vi "WSVCAP SHL FPGA TL Top Level.vi"() -> ()   [LabVIEW 2017]
uses:
  Type Defs/WSVCAP SHL State.ctl
  Type Defs/WSVCAP SHL Transaction Enum.ctl
  Type Defs/WSVCAP SHL Communication Loop State.ctl
  Type Defs/WSVCAP SHL FIFO Operation Enum.ctl
  Type Defs/WSVCAP SHL Operation Step Enum.ctl
  Type Defs/WSVCAP SHL Procedure Step Enum.ctl
  Type Defs/WSVCAP SHL Transaction Step Enum.ctl
  <vilib>/Platform/TimedLoop/XDataNode/timing_clust.ctl
  <vilib>/Platform/TimedLoop/XDataNode/nitl_modes.ctl
  <vilib>/Platform/TimedLoop/XDataNode/wakeup.ctl
  WSVCAP Shell FPGA Low Level/WSVCAP SHL FPGA LL RFFE Debug Global.vi
  WSVCAP Shell FPGA Low Level/WSVCAP SHL FPGA LL I2C Debug Global.vi
  <vilib>/Platform/TimedLoop/XDataNode/XDataNode.xnode
  <vilib>/Platform/TimedLoop/XDataNode/XDNodeRunTimeDep.lvlib
panel:
  in  "UUT Set":u8=8
  in  "Stop Cycle":bool
  out "Cycle Count":u64
  in  "Socket Mask":u64=1 format="%012x"
  in  "Display CH (1-48)":i32=1 min=1 max=48 step=1
  out "Status":i32
  out "Read Data":u64
  in  "Transaction":T1
  in  "Bytes to Write":u8=8
  in  "Sub Address":u8=1 format="%02x"
  in  "Ack Read Status":bool
  out "Read Status Flag":bool
  in  "Exit":bool
  out "Waveform Chart":cluster{i16, i16, i16, i16}(graph)
  in  "Wait Ticks":u32=20
  in  "Slave Address":u8=1 format="%02x"
  in  "Bytes to Read":u8=8
  in  "Start":bool
  in  "Cmd":T2
  in  "Ack Read":bool
  out "Read Flag":bool
  in  "Write Flag":bool
  in  "Write Data":u64
  # "Control"
  # "Configuration Parameters"
  # "Host Data Transfer"
  # "Command Type"
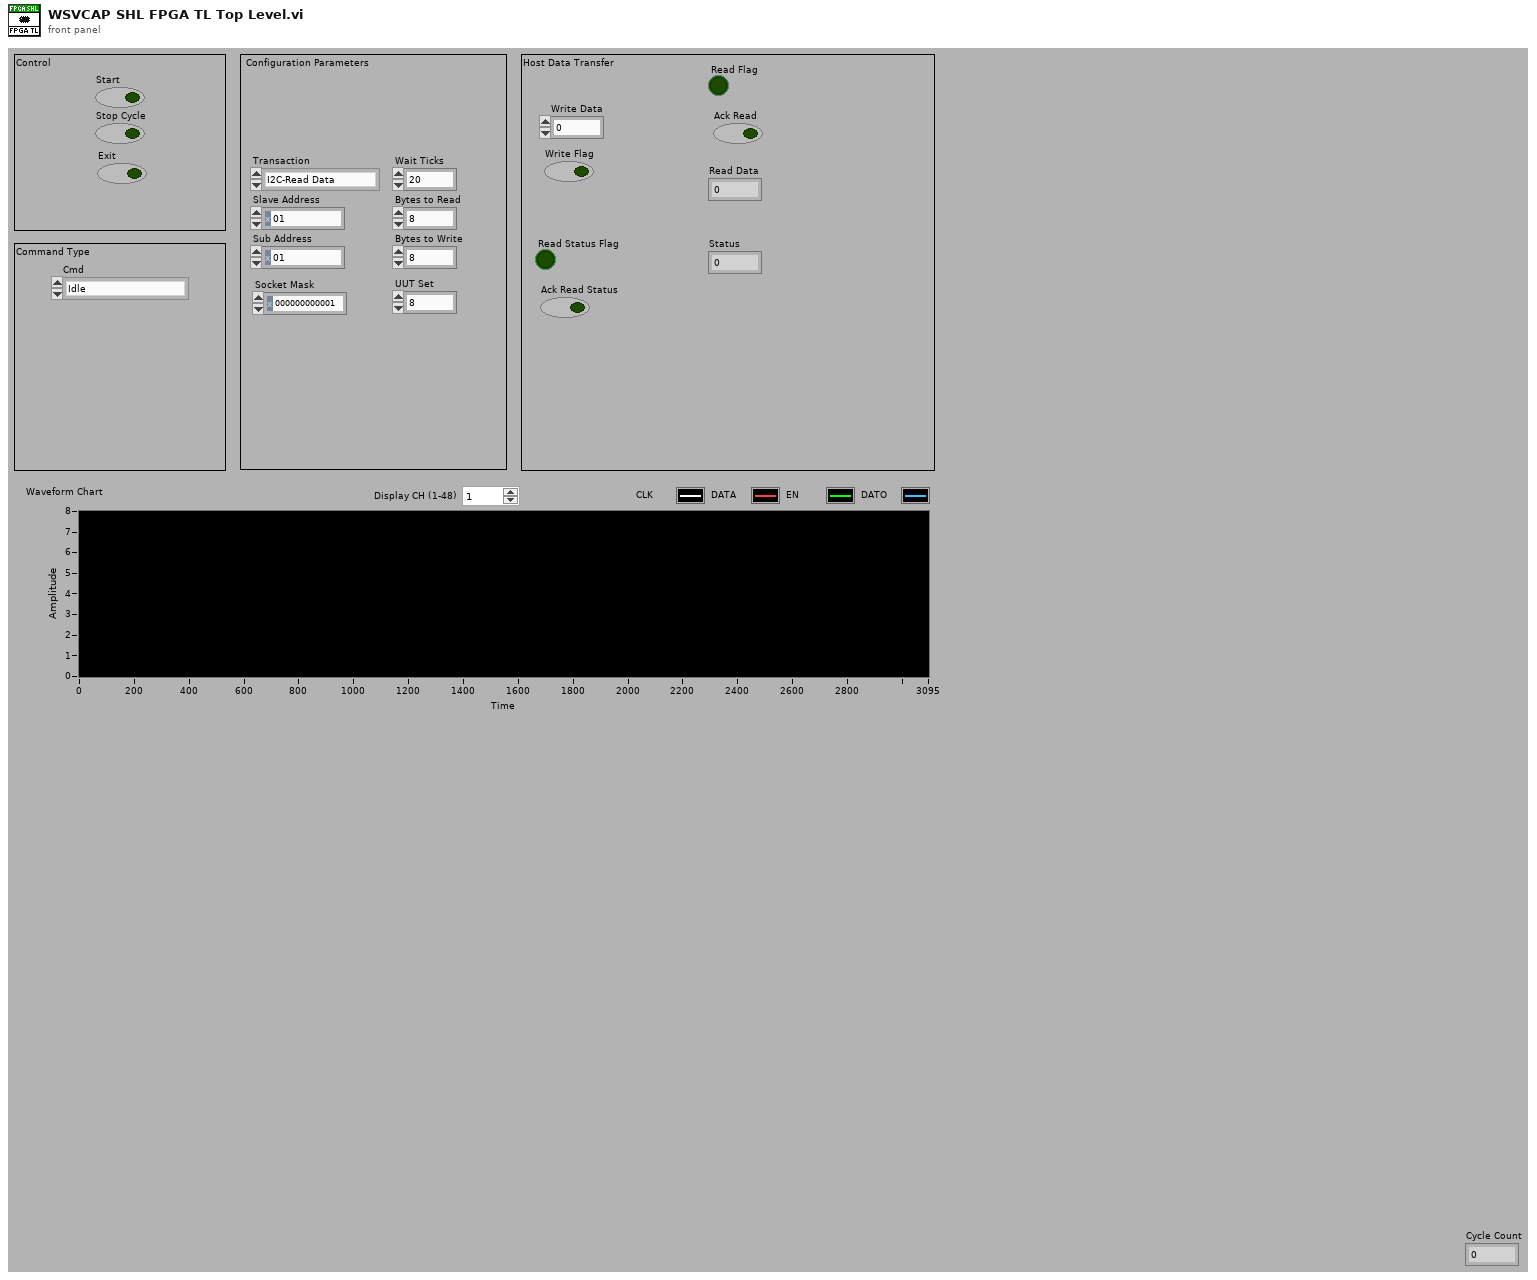
[diagram p1: front panel]
types:
  T1 = typedef "WSVCAP SHL Transaction Enum.ctl" = enum16{"I2C-Read Data", "I2C-Write Data", "RFFE-Ext Write", "RFFE-Ext Read"}
  T2 = typedef "WSVCAP SHL State.ctl" = enum8{"Idle", "Transfer Data"}
  T3 = typedef "WSVCAP SHL Communication Loop State.ctl" = enum8{"Idle", "Initialize", "Pre-Transmission", "Transmit Data", "Post Transmition", "Operation Complete"}
  T4 = typedef "WSVCAP SHL FIFO Operation Enum.ctl" = enum16{"Create FIFO/Memory", "Get Write FIFO Status", "Get Read FIFO Status", "Put Element in Write", "Put Element in Read", "Get Element from Write", "Get Element from Read"}
  T5 = typedef "WSVCAP SHL Procedure Step Enum.ctl" = enum16{"I2C Start/Stop - 1: Set Clock Low", "I2C Start/Stop - 2: Wait", "I2C Start/Stop - 3: Set Data I", "I2C Start/Stop - 4: Wait", "I2C Start/Stop - 5: Set Clock High", "I2C Start/Stop - 6: Wait", "I2C Start/Stop - 7: Set Data II", "I2C Start/Stop - 8: Wait", "I2C Start/Stop - 9: Set Clock Low", "I2C Start/Stop - 10: Wait", "I2C Read ACK - 1: Set Clock High", "I2C Read ACK - 2: Wait", "I2C Read ACK - 3: Read ACK Bit", "I2C Read ACK - 4: Wait", "I2C Read ACK - 5: Set Clock Low", "I2C Read ACK - 6: Wait", "I2C Write ACK - 1: Write ACK Bit", "I2C Write ACK - 2: Wait", "I2C Write ACK - 3: Set Clock High", "I2C Write ACK - 4: Wait", "I2C Write ACK - 5: Set Clock Low", "I2C Write ACK - 6: Wait", "I2C Write ACK - 7: Set Data Low", "I2C Send Add - 1: Reset Bits Remaining", "I2C Send Add - 2: Set Data Bit", "I2C Send Add - 3: Wait", "I2C Send Add - 4: Set Clock High", "I2C Send Add - 5: Wait", "I2C Send Add - 6: Set Clock Low", "I2C Send Add - 7: Wait", "I2C Send Add - 8: Check Bits Remaining", "I2C Send Data - 1: Reset Bits Remaining", "I2C Send Data - 2: Load Write Bit from FIFO", "I2C Send Data - 3: Set Data Bit", "I2C Send Data - 4: Wait", "I2C Send Data - 5: Set Clock High", "I2C Send Data - 6: Wait", "I2C Send Data - 7: Set Clock Low", "I2C Send Data - 8: Wait", "I2C Send Data - 9: Check Bits Remaining", "I2C Receive Data - 1: Reset Bits Remaining", "I2C Receive Data - 2: Wait", "I2C Receive Data - 3: Set Clock High", "I2C Receive Data - 4: Wait", "I2C Receive Data - 5: Read Data Bit", "I2C Receive Data - 6: Wait", "I2C Receive Data - 7: Set Clock Low", "I2C Receive Data - 8: Wait", "I2C Receive Data - 9: Check Bits Remaining", "RFFE Send SSC - 1:Set Low", "RFFE Send SSC - 2:Wait", "RFFE Send SSC - 3:Set SDA High", "RFFE Send SSC - 4:Wait", "RFFE Send SSC - 5:Set SDA Low", "RFFE Send SSC - 6:Wait", "RFFE Send Data - 1:Set SCL High", "RFFE Send Data - 2:Wait", "RFFE Send Data - 3:Set SCL Low", "RFFE Send Data - 4:Wait", "RFFE Send Data - 5:Set SCL High (P)", "RFFE Send Data - 6:Wait", "RFFE Send Data - 7:Set SCL Low (P)", "RFFE Send Data - 8:Wait", "RFFE Send Data - 9:Set SCL High (BP)", "RFFE Send Data - 10:Wait", "RFFE Send Data - 11:Set SCL Low (BP)", "RFFE Send Data - 12:Wait", "RFFE Receive Data - 1:Set SCL High", "RFFE Receive Data - 2:Wait", "RFFE Receive Data - 3:Set SCL Low", "RFFE Receive Data - 4:Wait", "RFFE Receive Data - 5:Set SCL High (BP)", "RFFE Receive Data - 6:Wait", "RFFE Receive Data - 7:Set SCL Low (BP)", "RFFE Receive Data - 8:Wait", "RFFE Wait CMD Delay - 1:Wait", "RFFE Clear Lines - 1:Clear"}
  T6 = typedef "WSVCAP SHL Operation Step Enum.ctl" = enum16{"I2C Send Slave Add - A: Send Start Sequence", "I2C Send Slave Add - B: Load Address Byte", "I2C Send Slave Add - C: Send Address Byte", "I2C Send Slave Add - D: Read Slave ACK", "I2C Send Sub Add - A: Load Sub Address", "I2C Send Sub Add - B: Send Address Byte", "I2C Send Sub Add - C: Read Slave ACK", "I2C Send Data - A: Get Byte from FIFO", "I2C Send Data - B: Send Data Byte", "I2C Send Data - C: Read Slave ACK", "I2C Send Data - D: Send Stop Sequence", "I2C Read Data - A: Load Bytes to Read", "I2C Read Data - B: Receive Byte", "I2C Read Data - C: Write Master ACK", "I2C Read Data - D: Send Stop Sequence", "RFFE Read Data - A: Send SSC", "RFFE Read Data - B: Send CMD Frame", "RFFE Read Data - C: Receive Byte", "RFFE Write Data - A: Send SSC", "RFFE Write Data - B: Send Data", "RFFE Write Data - C: Wait CMD Delay", "RFFE Write Data - D: Clear Lines"}
  T7 = typedef "WSVCAP SHL Transaction Step Enum.ctl" = enum16{"I2C Write - I:Send Slave Address", "I2C Write - II:Send Sub Address", "I2C Write - III:Send Data Bytes", "I2C Read - I:Send Slave Address (W)", "I2C Read - II:Send Sub Address", "I2C Read - III:Send Slave Address (R)", "I2C Read - IV:Read Data Bytes", "RFFE Ext Write - I.Write Data", "RFFE Ext Read - I:Read Data"}
  T8 = typedef "XDNodeRunTimeDep.lvlib/timing_clust.ctl" = cluster{"Expected End [f-1]":u64, "Actual End [f-1]":u64, "Finished Late? [f-1]":bool, "Expected End [i-1]":u64, "Actual End [i-1]":u64, "Finished Late? [i-1]":bool, "Expected Start [i]":u64, "Actual Start [i]":u64, "Expected Start [f]":u64, "Actual Start [f]":u64, "Source Name":string, "Structure Name":string, "Period":i64, "Deadline":i64, "Offset":i64, "Start":i64, "Priority":i32, "Timeout":i32, "Mode":T9, "Wakeup Reason":T10, "Error":errorcluster, "Source Type":string, "Secondary Source Type":string, "Global End Time":u64, "Global Start Time":u64, "Frame Duration":u64, "Iteration Duration":u64, "Assigned CPU":i32, "I/O Scan Engine Mode":u32}
  T9 = typedef "XDNodeRunTimeDep.lvlib/nitl_modes.ctl" = enum32{"No Change", "Process missed periods, maintain original phase", "Discard missed periods, maintain original phase", "Process missed periods, ignore original phase", "Discard missed periods, ignore original phase"}
  T10 = typedef "XDNodeRunTimeDep.lvlib/wakeup.ctl" = enum32{"Normal", "Aborted", "Asynchronous wakeup", "Timing source error", "Timed loop error", "Timeout"}
  T11 = typedef "WSVCAP SHL Transaction Cluster.ctl" = cluster{"Transaction":T1, "Write Byte":u8, "Write Bits Remaining":u8, "Read Bits Remaining":u8, "Read Bytes Remaining":u8, "Wait Ticks Remaining":u32, "Slave Address":u8, "Bytes to Read":u8, "Bytes to Write":u8, "Sub Address":u8, "Socket Mask":u64, "Write CMD [1-4]":u8, "Write Bit Index [0-39]":u8, "CMD Delay (Ticks)":u32, "Commands per Cycle [1-4]":u8, "CMD Length [1-48]":u8, "Cycle Count":u64, "Cycle Mode":bool, "CMD 1 Length (Bits)":u8, "CMD 2 Length (Bits)":u8, "CMD 3 Length (Bits)":u8, "CMD 4 Length (Bits)":u8, "CMD 1 Delay (Ticks)":u32, "CMD 2 Delay (Ticks)":u32, "CMD 3 Delay (Ticks)":u32, "CMD 4 Delay (Ticks)":u32, "CMD 1":u64, "CMD 2":u64, "CMD 3":u64, "CMD 4":u64, "Cycle CMD":u64, "Transaction Step":T7, "Operation Step":T6, "Procedure Step":T5, "Start Operation":bool, "Start Procedure":bool, "Procedure":T12, "Wait Ticks":u32, "UUT Set (0/1)":u8}
  T12 = typedef "WSVCAP SHL Procedure Enum.ctl" = enum16{"None", "I2C-Send Start/Stop Sequence", "I2C-Send Address Byte", "I2C-Send Data Byte", "I2C-Read ACK", "I2C-Receive Byte", "I2C-Write ACK", "RFFE-Clear Lines", "RFFE-Send SSC", "RFFE-Send Data", "RFFE-Receive Data", "RFFE-Wait CMD Delay"}
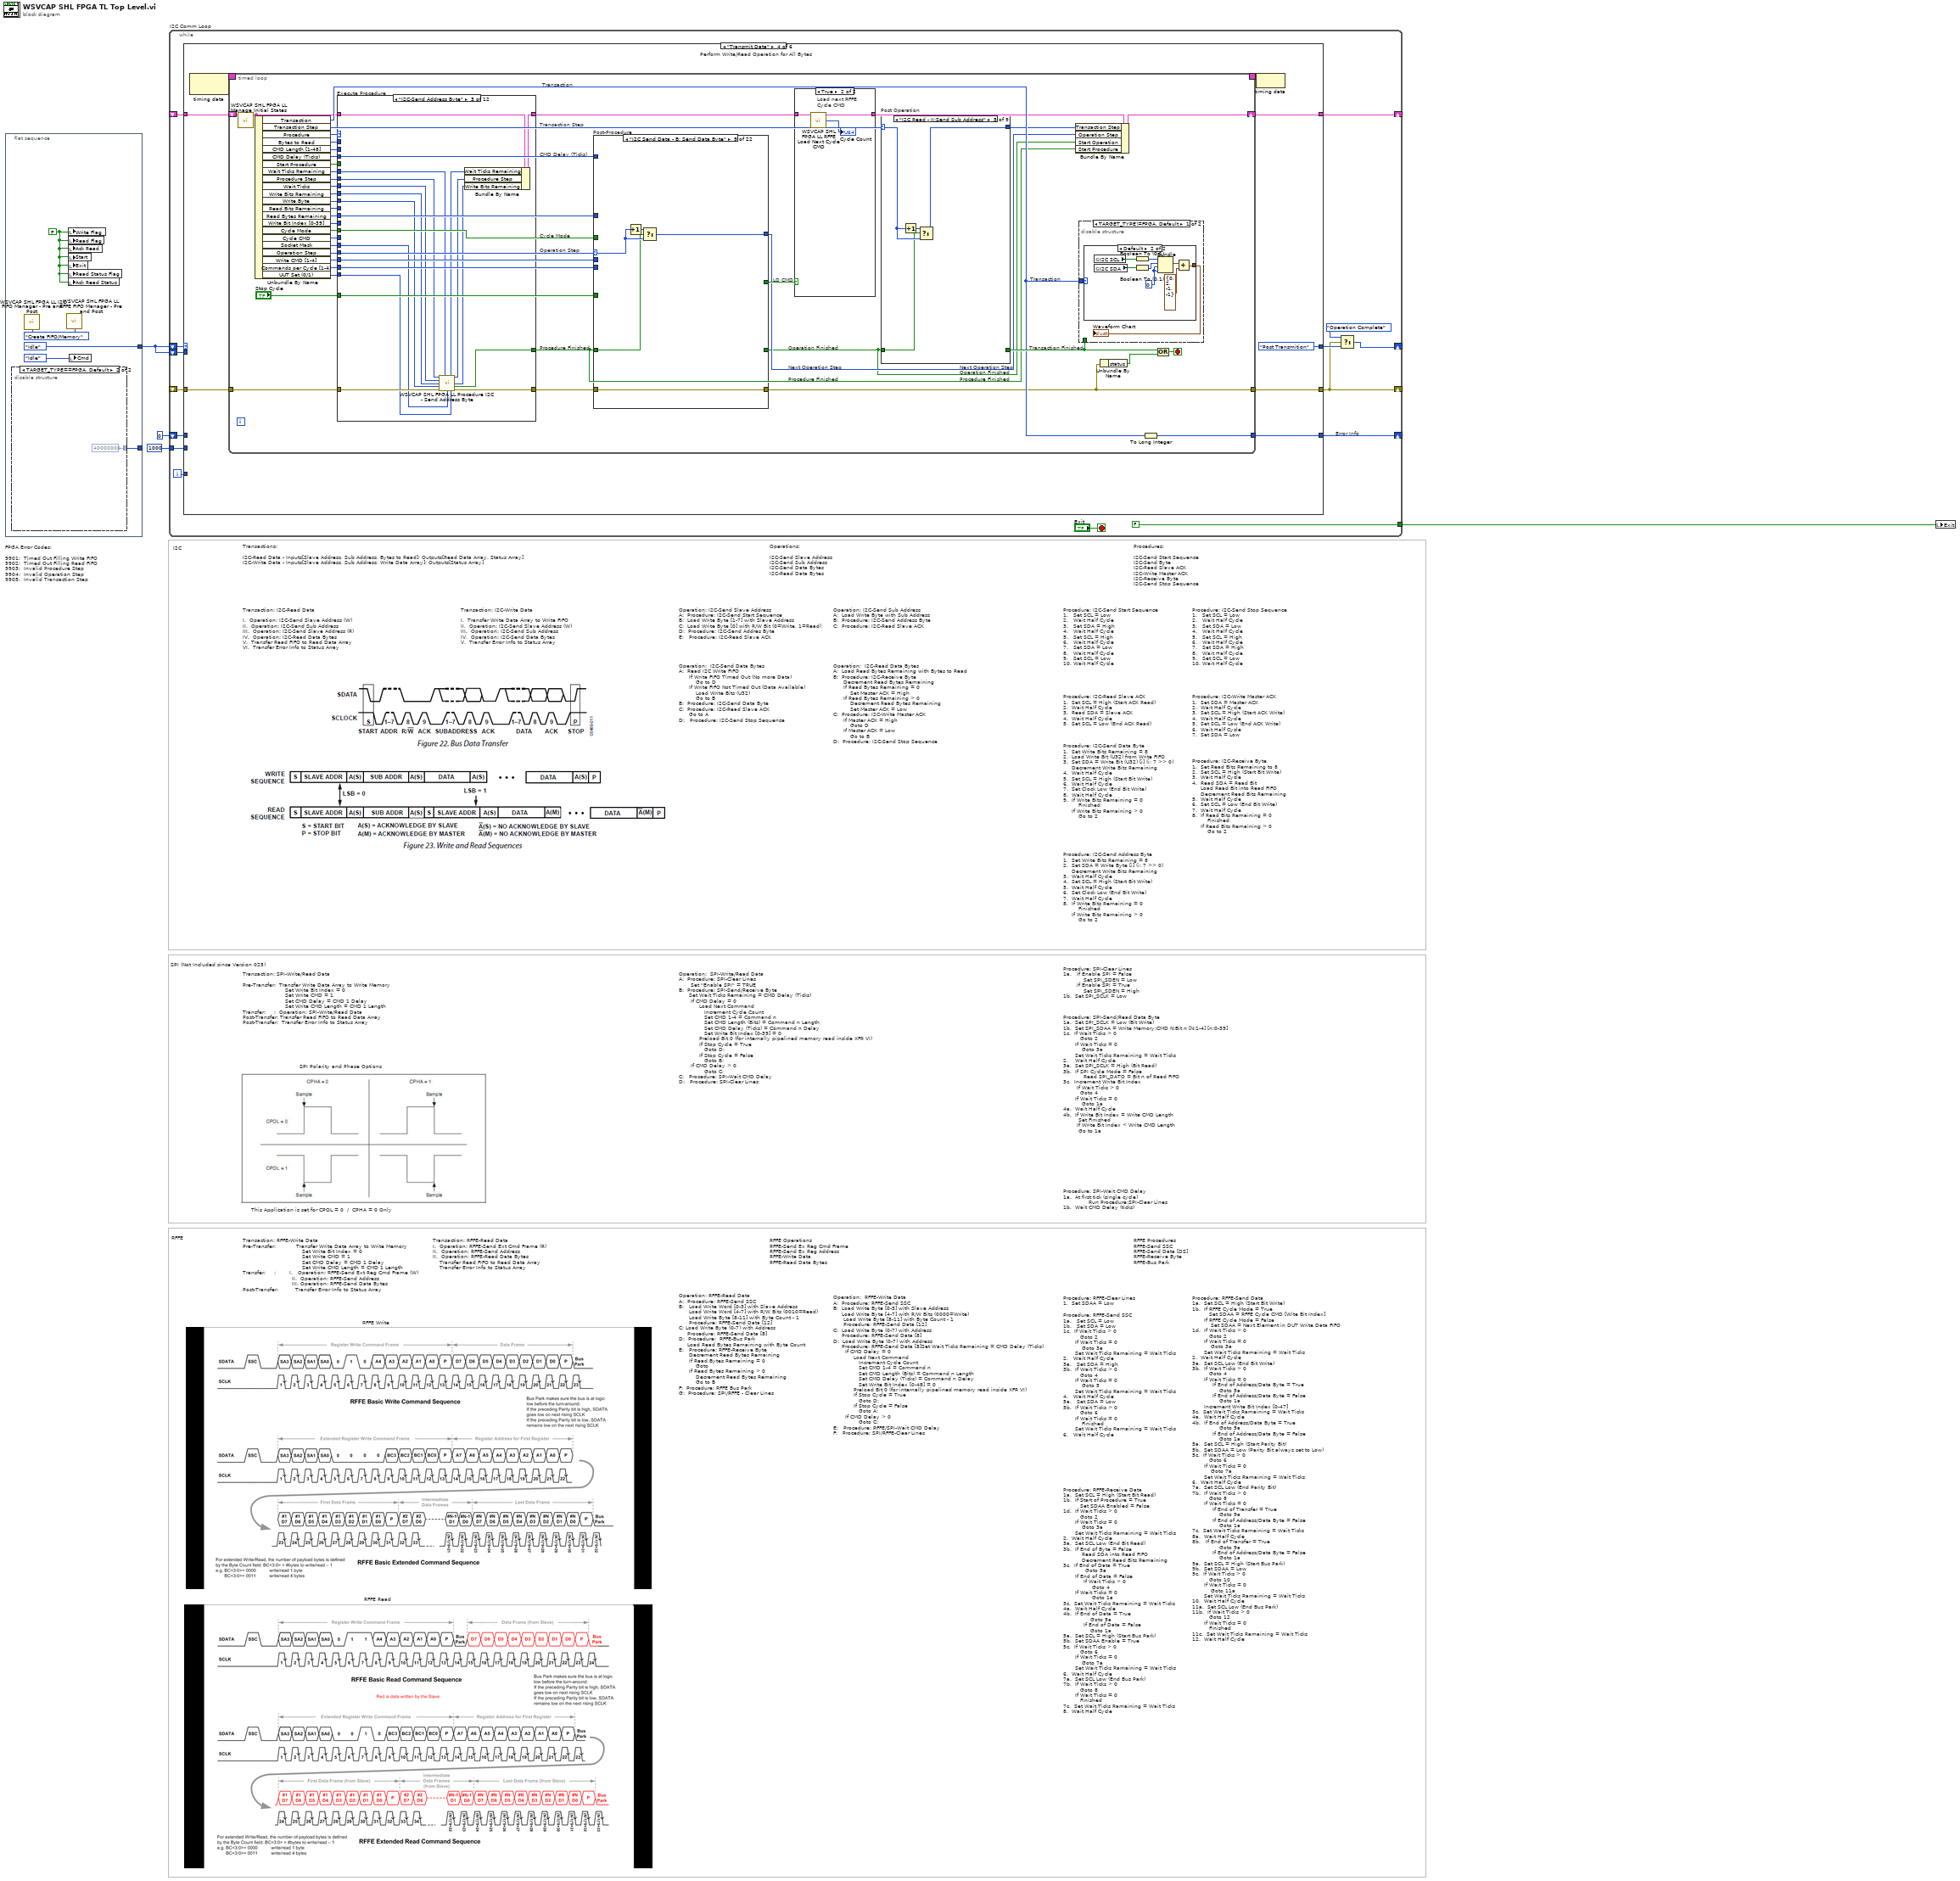
[diagram p0: block diagram]
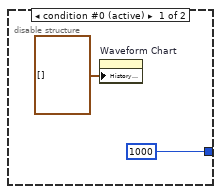
[diagram p2: hidden frame]
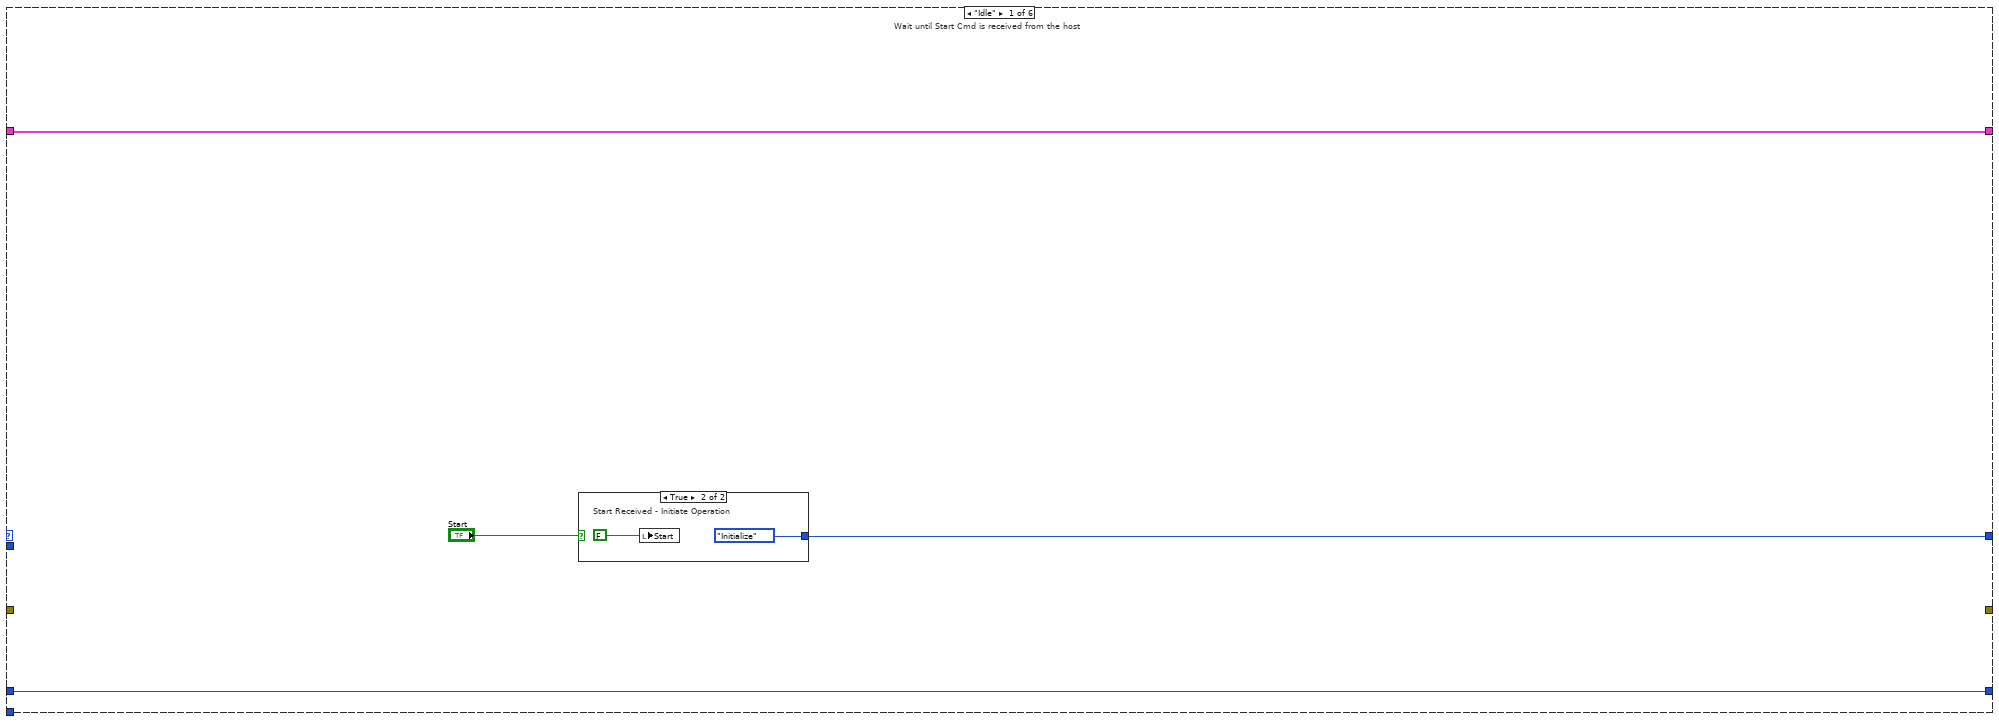
[diagram p3: hidden frame]
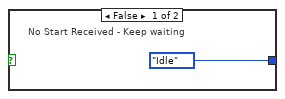
[diagram p4: hidden frame]
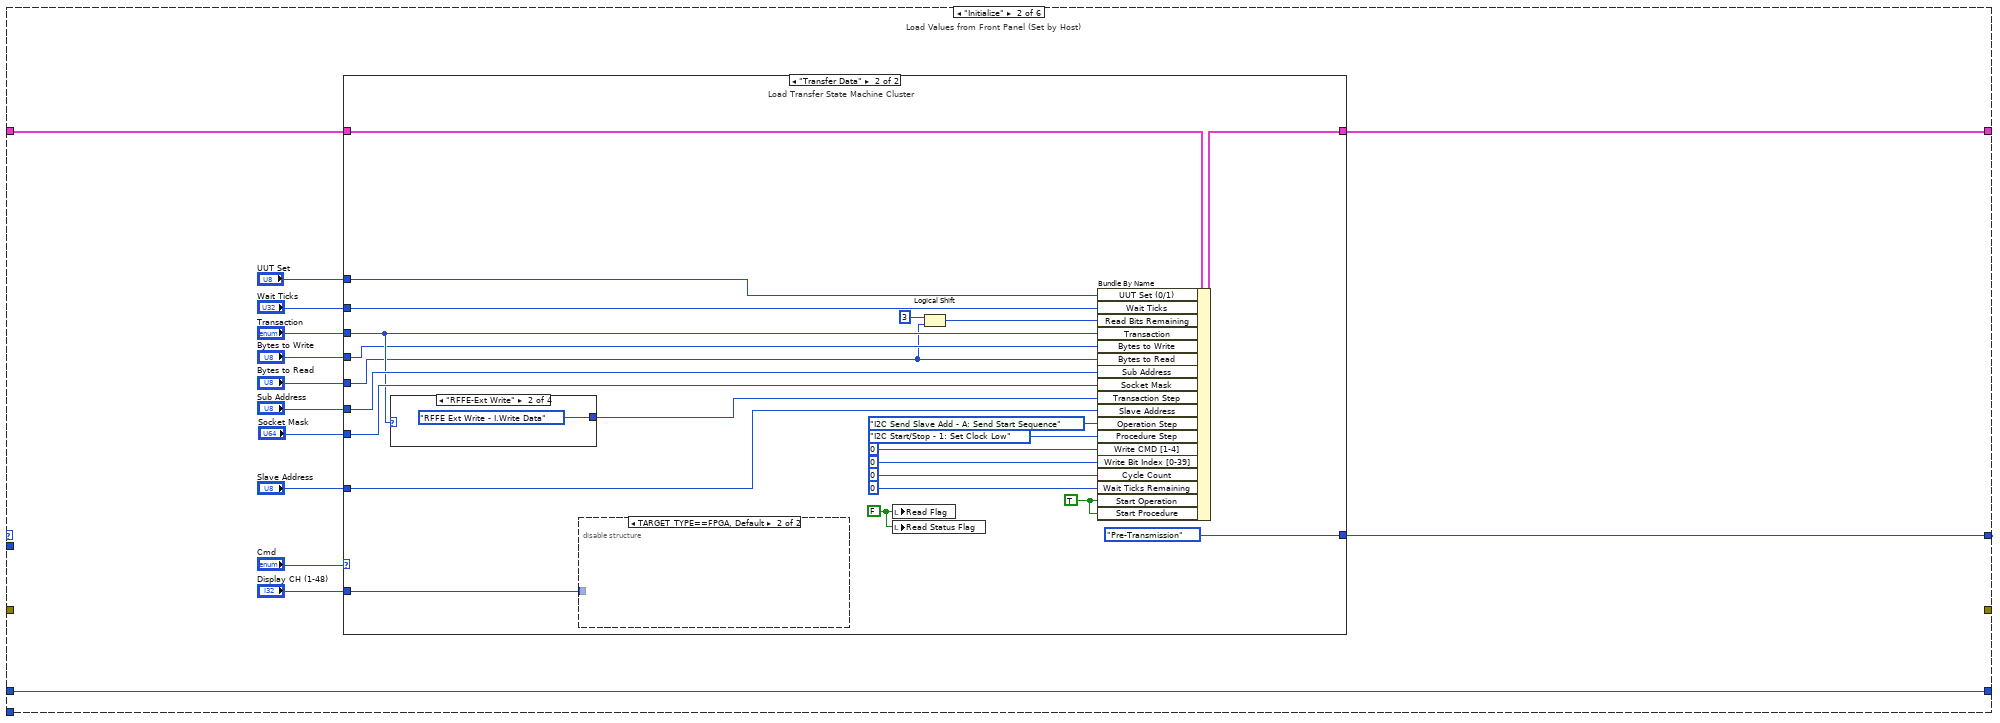
[diagram p5: hidden frame]
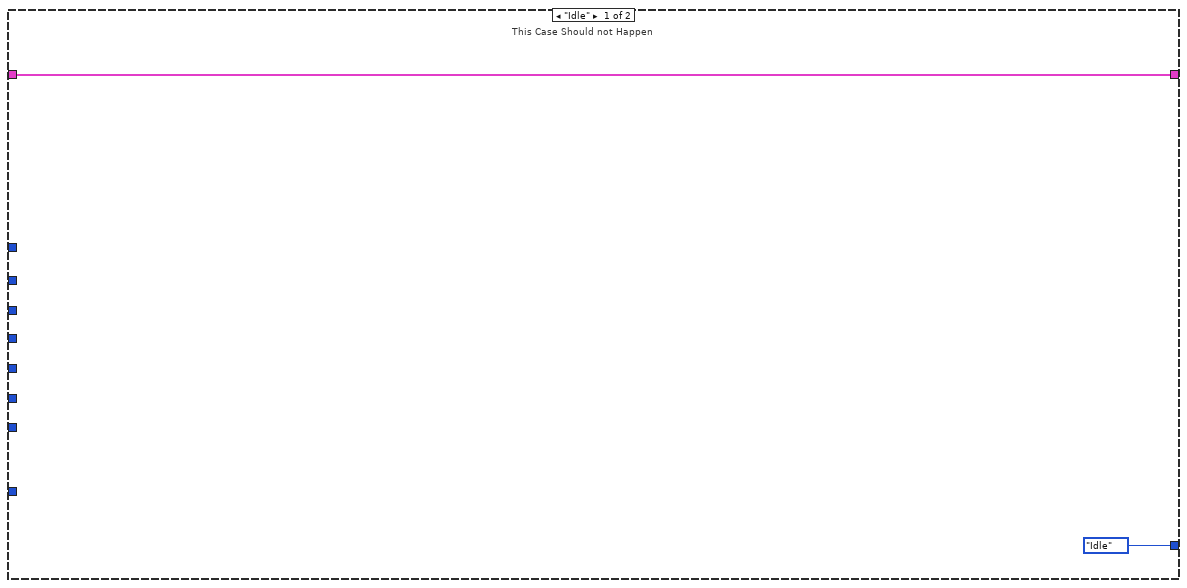
[diagram p6: hidden frame]
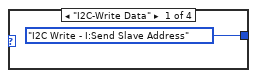
[diagram p7: hidden frame]
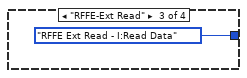
[diagram p8: hidden frame]
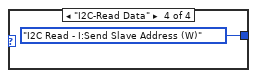
[diagram p9: hidden frame]
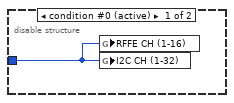
[diagram p10: hidden frame]
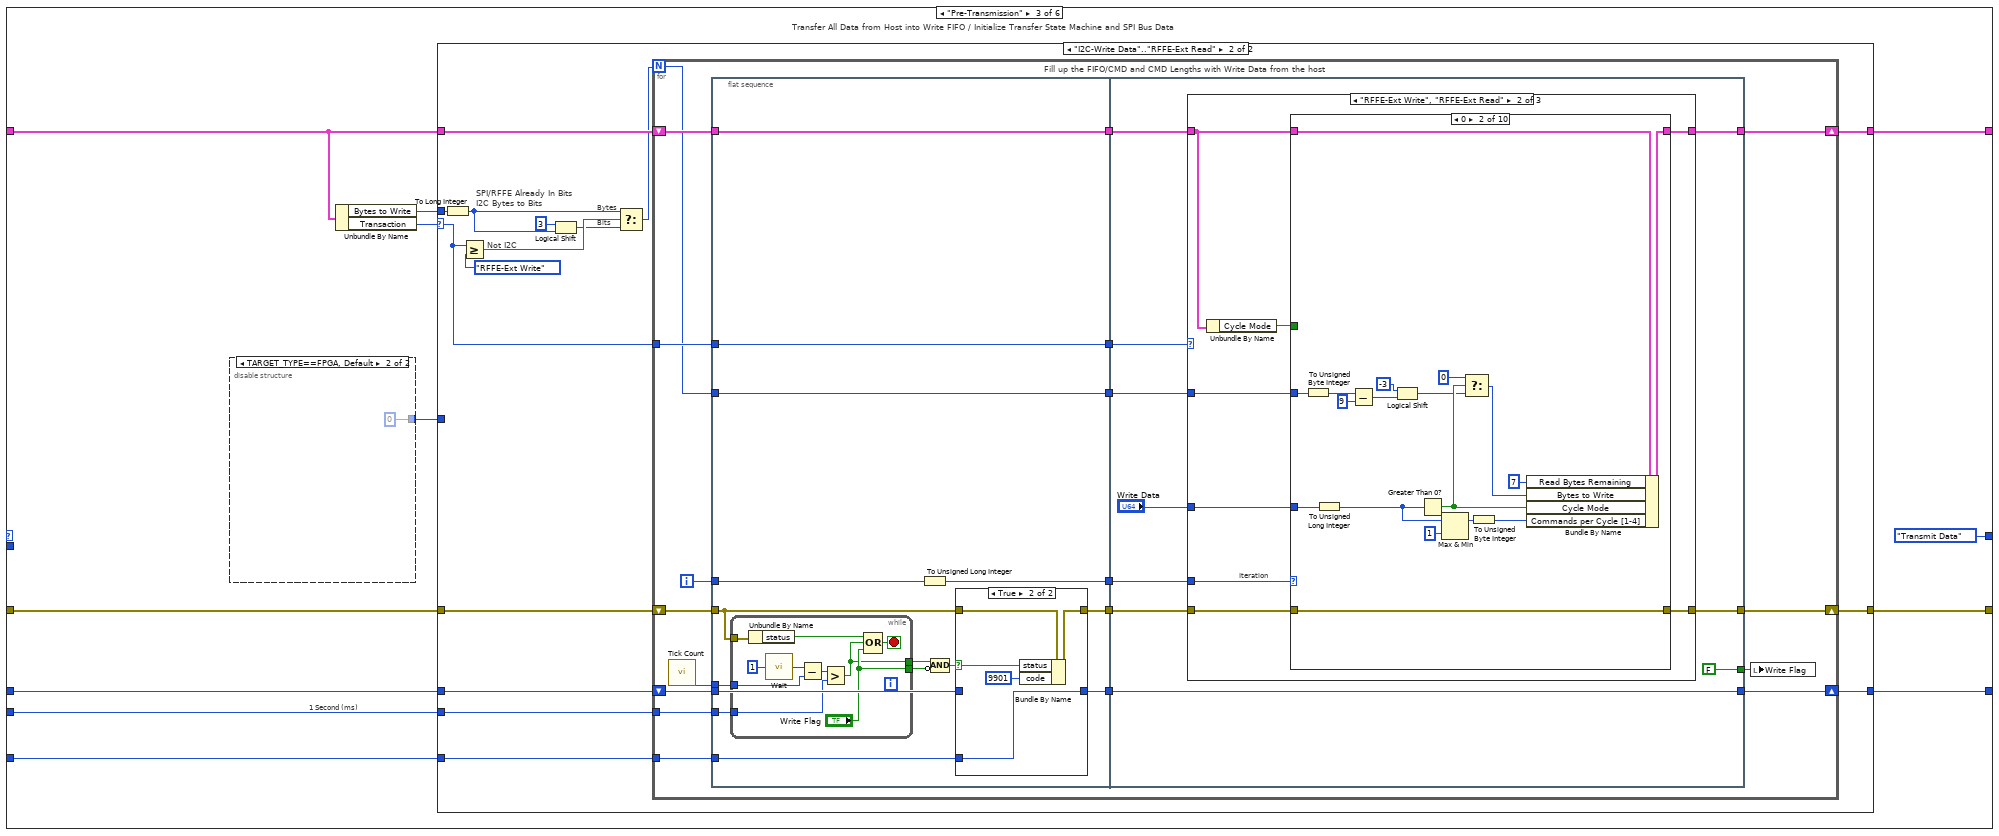
[diagram p11: hidden frame]
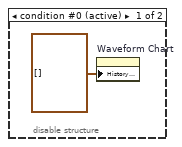
[diagram p12: hidden frame]
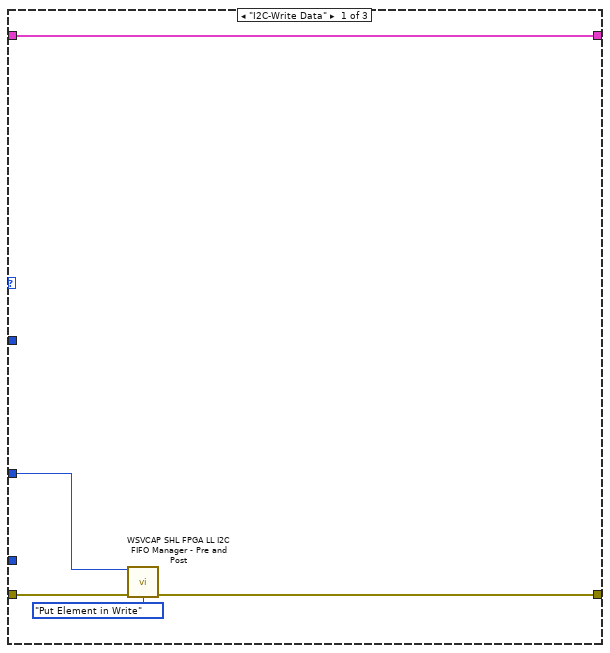
[diagram p15: hidden frame]
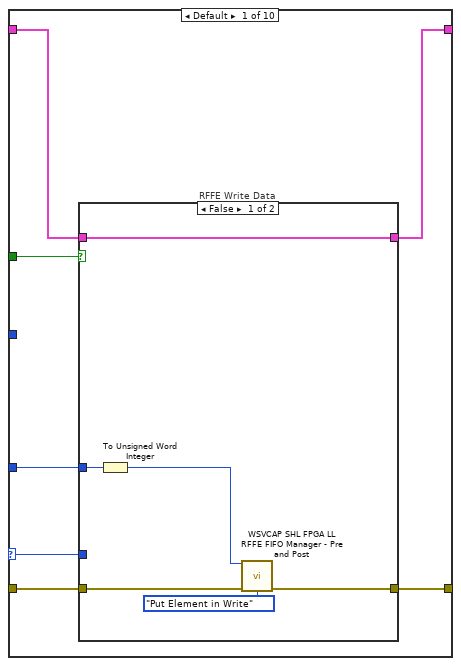
[diagram p16: hidden frame]
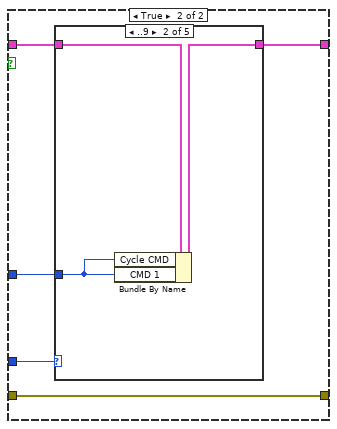
[diagram p17: hidden frame]
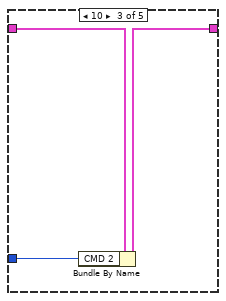
[diagram p19: hidden frame]
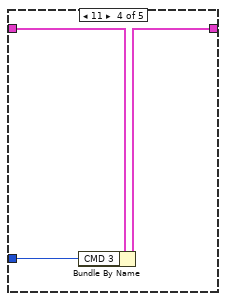
[diagram p20: hidden frame]
diagram:
  # "RFFE"
  # "SPI (Not Included since Version 025)"
  # "I2C"
  # "Procedure: RFFE-Receive Data\n1a.  Set SCL = High (Start Bit Read)\n1b.  If Start of Procedure = True\n          Set SDAA Enabled = False\n1d.  If Wait Ticks > 0\n          Goto 2\n       If Wait Ticks = 0 \n           Goto 3a\n       Set Wait Ticks Ramaining = Wait Ticks\n2.  Wait Half Cycle\n3a.  Set SCL Low (End Bit Read)\n3b.  If End of Byte = False\n           Read SDA into Read FIFO\n           Decrement Read Bits Remaining\n3c.  If End of Data = True\n             Goto 5a\n       If End of Data = False\n            If Wait Ticks > 0\n                 Goto 4\n       If Wait Ticks = 0         \n                 Goto 1a\n3c.  Set Wait Ticks Ramaining = Wait Ticks     \n4a.  Wait Half Cycle\n4b.  If End of Data = True\n                Goto 5a\n            If End of Data = False\n                Goto 1a\n5a.  Set SCL = High (Start Bus Park)\n5b.  Set SDAA Enable = True\n5c.  If Wait Ticks > 0\n          Goto 6\n       If Wait Ticks = 0 \n           Goto 7a\n       Set Wait Ticks Ramaining = Wait Ticks\n6.  Wait Half Cycle\n7a.  Set SCL Low (End Bus Park)\n7b.  If Wait Ticks > 0\n          Goto 8\n       If Wait Ticks = 0 \n          Finished\n7c.  Set Wait Ticks Ramaining = Wait Ticks\n8.  Wait Half Cycle"
  # "Procedure: RFFE-Send Data\n1a.  Set SCL = High (Start Bit Write)\n1b.  If RFFE Cycle Mode = True\n          Set SDAA = RFFE Cycle CMD [Wite Bit Index]\n       If RFFE Cycle Mode = False\n           Set SDAA = Next Element in DUT Write Data FIFO\n1d.  If Wait Ticks > 0\n          Goto 2\n       If Wait Ticks = 0 \n           Goto 3a\n       Set Wait Ticks Ramaining = Wait Ticks\n2.  Wait Half Cycle\n3a.  Set SCL Low (End Bit Write)\n3b.  If Wait Ticks > 0\n          Goto 4\n       If Wait Ticks = 0 \n            If End of Address/Data Byte = True\n                Goto 5a\n            If End of Address/Data Byte = False\n                Goto 1a\n       Increment Write Bit Index [0-47]\n3c.  Set Wait Ticks Ramaining = Wait Ticks     \n4a.  Wait Half Cycle\n4b.  If End of Address/Data Byte = True\n                Goto 5a\n            If End of Address/Data Byte = False\n                Goto 1a\n5a.  Set SCL = High (Start Parity Bit)\n5b.  Set SDAA = Low (Parity Bit always set to Low)\n5c.  If Wait Ticks > 0\n          Goto 6\n       If Wait Ticks = 0 \n           Goto 7a\n       Set Wait Ticks Ramaining = Wait Ticks\n6.  Wait Half Cycle\n7a.  Set SCL Low (End Parity Bit)\n7b.  If Wait Ticks > 0\n          Goto 8\n       If Wait Ticks = 0 \n            If End of Transfer = True\n                Goto 9a\n            If End of Address/Data Byte = False\n                Goto 1a\n7c.  Set Wait Ticks Ramaining = Wait Ticks\n8a.  Wait Half Cycle\n8b.   If End of Transfer = True\n                Goto 9a\n            If End of Address/Data Byte = False\n                Goto 1a\n9a.  Set SCL = High (Start Bus Park)\n9b.  Set SDAA = Low\n9c.  If Wait Ticks > 0\n          Goto 10\n       If Wait Ticks = 0 \n           Goto 11a\n       Set Wait Ticks Ramaining = Wait Ticks\n10.  Wait Half Cycle\n11a.  Set SCL Low (End Bus Park)\n11b.  If Wait Ticks > 0\n          Goto 12\n       If Wait Ticks = 0 \n          Finished\n11c.  Set Wait Ticks Ramaining = Wait Ticks\n12.  Wait Half Cycle"
  # "Procedure: RFFE-Send SSC\n1a.   Set SCL = Low\n1b.   Set SDA = Low\n1c.  If Wait Ticks > 0\n          Goto 2\n       If Wait Ticks = 0 \n           Goto 3a\n       Set Wait Ticks Ramaining = Wait Ticks\n2.   Wait Half Cycle\n3a.   Set SDA = High\n3b.  If Wait Ticks > 0\n          Goto 4\n       If Wait Ticks = 0 \n           Goto 5\n       Set Wait Ticks Ramaining = Wait Ticks\n4.   Wait Half Cycle\n5a.   Set SDA = Low\n5b.  If Wait Ticks > 0\n          Goto 6\n       If Wait Ticks = 0 \n           Finished\n       Set Wait Ticks Ramaining = Wait Ticks\n6.   Wait Half Cycle"
  # "Procedure: SPI-Clear Lines\n1a.   If Enable SPI = False\n            Set SPI_SDEN = Low\n        If Enable SPI = True\n            Set SPI_SDEN = High\n1b.  Set SPI_SCLK = Low"
  # "Procedure: RFFE-Clear Lines\n1.  Set SDAA = Low"
  # "Operation:  RFFE-Write Data\nA:  Procedure: RFFE-Send SSC\nB:  Load Write Byte [0-3] with Slave Address\n     Load Write Byte [4-7] with R/W Bits (0000=Write)\n      Load Write Byte [8-11] with Byte Count - 1\n      Procedure: RFFE-Send Data [12]\nC:  Load Write Byte (0-7) with Address\n     Procedure: RFFE-Send Data [8]\nD:  Load Write Byte (0-7) with Address\n     Procedure: RFFE-Send Data [8]Set Wait Ticks Remaining = CMD Delay (Ticks)\n       If CMD Delay = 0\n            Load Next Command\n               Increment Cycle Count\n               Set CMD 1-4 = Command n\n               Set CMD Length (Bits) = Command n Length\n               Set CMD Delay (Ticks) = Command n Delay\n               Set Write Bit Index [0-48] = 0\n            Preload Bit 0 (for internally pipelined memory read inside XFR VI)\n            If Stop Cycle = True\n               Goto D:\n            If Stop Cycle = False\n               Goto A:\n       If CMD Delay > 0\n               Goto C:\nE:   Procedure: RFFE/SPI-Wait CMD Delay          \nF:   Procedure: SPI/RFFE-Clear Lines"
  # "Operation: RFFE-Read Data\nA:  Procedure: RFFE-Send SSC\nB:   Load Write Word [0-3] with Slave Address\n      Load Write Word [4-7] with R/W Bits (0010=Read)\n      Load Write Byte [8-11] with Byte Count - 1\n      Procedure: RFFE-Send Data [12]\nC: Load Write Byte (0-7) with Address\n     Procedure: RFFE-Send Data [8]\nD:  Procedure:  RFFE-Bus Park\n     Load Read Bytes Remaining with Byte Count\nE:   Procedure: RFFE-Receive Byte\n      Decrement Read Bytes Remaining\n      If Read Bytes Remaining = 0\n          Goto\n      If Read Bytes Remaining > 0\n          Decrement Read Bytes Remaining\n          Go to B\nF:  Procedure: RFFE Bus Park\nG:  Procedure: SPI/RFFE - Clear Lines"
  # "RFFE Write"
  # "RFFE Read"
  # "Transaction: RFFE-Write Data\nPre-Transfer:            Transfer Write Data Array to Write Memory\n                                   Set Write Bit Index = 0\n                                   Set Write CMD = 1\n                                   Set CMD Delay = CMD 1 Delay\n                                   Set Write CMD Length = CMD 1 Length\nTransfer:     :        I.   Operation: RFFE-Send Ext Reg Cmd Frame (W)\n                             II.  Operation: RFFE-Send Address\n                             III. Operation: RFFE-Send Data Bytes\nPost-Transfer:          Transfer Error Info to Status Array"
  # "RFFE Procedures\nRFFE-Send SSC\nRFFE-Send Data [DS]\nRFFE-Receive Byte\nRFFE-Bus Park"
  # "Transaction: RFFE-Read Data\nI.  Operation: RFFE-Send Ext Cmd Frame (R)\nII.  Operation: RFFE-Send Address\nII.  Operation: RFFE-Read Data Bytes\n    Transfer Read FIFO to Read Data Array\n    Transfer Error Info to Status Array"
  # "RFFE Operations\nRFFE-Send Ex Reg Cmd Frame\nRFFE-Send Ex Reg Address\nRFFE-Write Data\nRFFE-Read Data Bytes"
  # "SPI Polarity and Phase Options"
  # "Procedure: SPI-Wait CMD Delay\n1a.  At first tick (single cycle)\n               Run Procedure:SPI-Clear Lines\n1b.  Wait CMD Delay (ticks)"
  # "This Application is set for CPOL = 0  /  CPHA = 0 Only"
  # "Procedure: SPI-Send/Read Data Byte\n1a.  Set SPI_SCLK = Low (Bit Write)\n1b.  Set SPI_SDAA = Write Memory:CMD N:Bit n [N:1-4] [n:0-39] \n1c.  If Wait Ticks > 0\n          Goto 2\n       If Wait Ticks = 0 \n           Goto 3a\n       Set Wait Ticks Ramaining = Wait Ticks\n2.    Wait Half Cycle\n3a.  Set SPI_SCLK = High (Bit Read)\n3b.  If SPI Cycle Mode = False\n            Read SPI_DATO = Bit n of Read FIFO            \n3c.  Increment Write Bit Index\n        If Wait Ticks > 0\n          Goto 4\n       If Wait Ticks = 0 \n           Goto 1a \n4a.  Wait Half Cycle\n4b.  If Write Bit Index = Write CMD Length\n         Set Finished\n        If Write Bit Index < Write CMD Length\n         Go to 1a"
  # "Operation:  SPI-Write/Read Data\nA:  Procedure: SPI-Clear Lines\n       Set \"Enable SPI\" = TRUE \nB:  Procedure: SPI-Send/Receive Byte\n      Set Wait Ticks Remaining = CMD Delay (Ticks)\n       If CMD Delay = 0\n            Load Next Command\n               Increment Cycle Count\n               Set CMD 1-4 = Command n\n               Set CMD Length (Bits) = Command n Length\n               Set CMD Delay (Ticks) = Command n Delay\n               Set Write Bit Index [0-39] = 0\n            Preload Bit 0 (for internally pipelined memory read inside XFR VI)\n            If Stop Cycle = True\n               Goto D:\n            If Stop Cycle = False\n               Goto B:\n       If CMD Delay > 0\n               Goto C:\nC:   Procedure: SPI-Wait CMD Delay          \nD:   Procedure: SPI-Clear Lines"
  # "FPGA Error Codes:\n\n9901:  Timed Out Filling Write FIFO\n9902:  Timed Out Filling Read FIFO\n9903:  Invalid Procedure Step\n9904:  Invalid Operation Step\n9905:  Invalid Transaction Step"
  # "Transaction: SPI-Write/Read Data\n\nPre-Transfer:  Transfer Write Data Array to Write Memory\n                         Set Write Bit Index = 0\n                         Set Write CMD = 1\n                         Set CMD Delay = CMD 1 Delay\n                         Set Write CMD Length = CMD 1 Length\nTransfer:     :  Operation: SPI-Write/Read Data\nPost-Transfer: Transfer Read FIFO to Read Data Array\nPost-Transfer:  Transfer Error Info to Status Array"
  # "Procedure: I2C-Send Address Byte\n1.  Set Write Bits Remaining = 8\n2.  Set SDA = Write Byte [i] (i: 7 >> 0)\n     Decrement Write Bits Remaining\n3.  Wait Half Cycle\n4.  Set SCL = High (Start Bit Write)\n5.  Wait Half Cycle\n6.  Set Clock Low (End Bit Write)\n7.  Wait Half Cycle\n8.  If Write Bits Remaining = 0\n         Finished\n     If Write Bits Remaining > 0\n         Go to 2"
  # "Procedure: I2C-Write Master ACK\n1.  Set SDA = Master ACK\n2.  Wait Half Cycle\n3.  Set SCL = High (Start ACK Write)\n4.  Wait Half Cycle\n5.  Set SCL = Low (End ACK Write)\n6.  Wait Half Cycle\n7.  Set SDA = Low"
  # "Procedure: I2C-Send Start Sequence\n1.   Set SCL = Low\n2.   Wait Half Cycle\n3.   Set SDA = High\n4.   Wait Half Cycle\n5.   Set SCL = High\n6.   Wait Half Cycle\n7.   Set SDA = Low\n8.   Wait Half Cycle\n9.   Set SCL = Low\n10. Wait Half Cycle"
  # "Procedure: I2C-Send Stop Sequence\n1.   Set SCL = Low\n2.   Wait Half Cycle\n3.   Set SDA = Low\n4.   Wait Half Cycle\n5.   Set SCL = High\n6.   Wait Half Cycle\n7.   Set SDA = High\n8.   Wait Half Cycle\n9.   Set SCL = Low\n10. Wait Half Cycle"
  # "Procedure: I2C-Read Slave ACK\n1.  Set SCL = High (Start ACK Read)\n2.  Wait Half Cycle\n3.  Read SDA = Slave ACK\n4.  Wait Half Cycle\n5.  Set SCL = Low (End ACK Read)"
  # "Procedure: I2C-Receive Byte\n1.  Set Read Bits Remaining to 8\n2.  Set SCL = High (Start Bit Write)\n3.  Wait Half Cycle\n4.  Read SDA = Read Bit\n     Load Read Bit into Read FIFO\n     Decrement Read Bits Remaining\n5.  Wait Half Cycle\n6.  Set SCL = Low (End Bit Write)\n7.  Wait Half Cycle\n8.  If Read Bits Remaining = 0\n         Finished\n     If Read Bits Remaining > 0\n         Go to 2"
  # "Procedure: I2C-Send Data Byte\n1.  Set Write Bits Remaining = 8\n2.  Load Write Bit (U32) from Write FIFO\n3.  Set SDA = Write Bit (U32) [i] (i: 7 >> 0)\n     Decrement Write Bits Remaining\n4.  Wait Half Cycle\n5.  Set SCL = High (Start Bit Write)\n6.  Wait Half Cycle\n7.  Set Clock Low (End Bit Write)\n8.  Wait Half Cycle\n9.  If Write Bits Remaining = 0\n         Finished\n     If Write Bits Remaining > 0\n         Go to 2"
  # "Operation:  I2C-Read Data Bytes\nA:  Load Read Bytes Remaining with Bytes to Read\nB:  Procedure: I2C-Receive Byte\n      Decrement Read Bytes Remaining\n      If Read Bytes Remaining = 0\n          Set Master ACK = High\n      If Read Bytes Remaining > 0\n          Decrement Read Bytes Remaining\n          Set Master ACK = Low\nC:  Procedure: I2C-Write Master ACK\n      If Master ACK = High\n          Goto D\n      If Master ACK = Low\n          Go to B\nD:  Procedure: I2C-Send Stop Sequence"
  # "Operation:  I2C-Send Data Bytes\nA:  Read I2C Write FIFO\n      If Write FIFO Timed Out (No more Data)\n          Go to D\n      If Write FIFO Not Timed Out (Data Available)\n          Load Write Bits (U32)\n          Go to B\nB:  Procedure: I2C-Send Data Byte\nC:  Procedure: I2C-Read Slave ACK\n      Go to A\nD:   Procedure: I2C-Send Stop Sequence"
  # "Operation: I2C-Send Sub Address\nA:  Load Write Byte with Sub Address\nB:  Procedure: I2C-Send Address Byte\nC:  Procedure: I2C-Read Slave ACK"
  # "Procedures:\n\nI2C-Send Start Sequence\nI2C-Send Byte\nI2C-Read Slave ACK\nI2C-Write Master ACK\nI2C-Receive Byte\nI2C-Send Stop Sequence"
  # "Transaction: I2C-Write Data\n\nI.  Transfer Write Data Array to Write FIFO\nII.  Operation: I2C-Send Slave Address (W)\nIII.  Operation: I2C-Send Sub Address\nIV.  Operation: I2C-Send Data Bytes\nV.  Transfer Error Info to Status Array"
  # "Transaction: I2C-Read Data\n\nI.  Operation: I2C-Send Slave Address (W)\nII.  Operation: I2C-Send Sub Address\nIII.  Operation: I2C-Send Slave Address (R)\nIV.  Operation: I2C-Read Data Bytes\nV.  Transfer Read FIFO to Read Data Array\nVI.  Transfer Error Info to Status Array"
  # "Transactions:\n\nI2C-Read Data - Inputs[Slave Address, Sub Address, Bytes to Read]; Outputs[Read Data Array, Status Array]\nI2C-Write Data - Inputs[Slave Address, Sub Address, Write Data Array]; Outputs[Status Array]"
  # "Operations:\n\nI2C-Send Slave Address\nI2C-Send Sub Address\nI2C-Send Data Bytes\nI2C-Read Data Bytes"
  # "Operation: I2C-Send Slave Address\nA:  Procedure: I2C-Send Start Sequence\nB:  Load Write Byte [1-7] with Slave Address\nC:  Load Write Byte [0] with R/W Bit (0=Write, 1=Read)\nD:  Procedure: I2C-Send Addres Byte\nE:   Procedure: I2C-Read Slave ACK"
  n1 = flat-sequence {
    tunnel: [WSVCAP_SHL_Communication_Loop_State."Idle" ("Action")] -> w3
    tunnel: [w6] -> _
    frame #0 {
      w5 = WSVCAP_SHL_FIFO_Operation_Enum."Create FIFO/Memory" ("Operation")
      w7 = FALSE ("Done")
      n2 = disable-structure shown="TARGET_TYPE==FPGA, Default" {
        disable-tunnel: [u32 1000 ("x-y") u32 40000000 ("x-y")] -> w6
        frame condition #0 (active) {
          n3 = property on="Waveform Chart" class="WFChart (strict)"("History Data"=cluster{i16, i16, i16, i16}[] []) -> ()  [unwired: 2 in, 2 out]
        }
        frame condition #1 {
        }
      }
      n4 = call "WSVCAP SHL FPGA LL I2C FIFO Manager - Pre and Post.vi"("Operation"=w5) -> ()  [unwired: 12 in, 3 out]
      n5 = call "WSVCAP SHL FPGA LL RFFE FIFO Manager - Pre and Post.vi"("Operation"=w5) -> ()  [unwired: 12 in, 3 out]
      n6 = local write "Write Flag"(w7) -> ()
      n7 = local write "Read Flag"(w7) -> ()
      n8 = local write "Ack Read"(w7) -> ()
      n9 = local write "Start"(w7) -> ()
      n10 = local write "Exit"(w7) -> ()
      n11 = local write "Read Status Flag"(w7) -> ()
      n12 = local write "Ack Read Status"(w7) -> ()
      n13 = local write "Cmd"(WSVCAP_SHL_State."Idle" ("SPI_CMD_DBG")) -> ()
    }
  }
  n14 = while "I2C Comm Loop" {
    shift-right: [w20] -> _
    shift-left: w3 -> [w27]
    shift-right: [w25] -> _
    shift-left: _ -> [w26]
    tunnel: [FALSE] -> w4
    shift-right: [w19] -> _
    shift-left: _ -> [w22]
    shift-left: w3 -> [w17]
    shift-right: [w16] -> _
    shift-left: 0 -> [w15]
    tunnel: u32 1000 ("x-y") -> [w14]
    i -> [w13]
    stop <- "Exit" stop-if-true
    # "Error Info"
    n15 = case shown="\"Transmit Data\"" w27 {
      tunnel: [w31 w47 WSVCAP_SHL_Communication_Loop_State."Transmit Data" ("Action") WSVCAP_SHL_Communication_Loop_State."Post Transmition" ("Action") WSVCAP_SHL_Communication_Loop_State."Operation Complete" ("Action") WSVCAP_SHL_Communication_Loop_State."Idle" ("Action")] -> w21
      tunnel: w26 -> [w28 w46 w81 w281 w670 w761]
      tunnel: [w28 w45 w80 w280 w669 w761] -> w25
      tunnel: [_ _ w83 w278 w677 _] -> w19
      tunnel: w22 -> [_ _ w88 w279 w678 w766]
      tunnel: w17 -> [_ _ _ _ _ w765]
      tunnel: [w29 w44 w84 w277 w674 _] -> w16
      tunnel: w15 -> [w29 w44 w85 _ w673 w763]
      tunnel: w14 -> [_ _ w87 _ w675 w762]
      tunnel: w13 -> [_ _ w86 _ _ _]
      frame "Idle" {
        # "Wait until Start Cmd is received from the host"
        n16 = case shown="True" "Start" {
          tunnel: [WSVCAP_SHL_Communication_Loop_State."Idle" ("Action") WSVCAP_SHL_Communication_Loop_State."Initialize" ("Action")] -> w31
          frame False {
            # "No Start Received - Keep waiting"
          }
          frame True {
            # "Start Received - Initiate Operation"
            n17 = local write "Start"(FALSE ("SPI_Start")) -> ()
          }
        }
      }
      frame "Initialize" {
        # "Load Values from Front Panel (Set by Host)"
        n18 = case shown="\"Transfer Data\"" "Cmd" {
          tunnel: [WSVCAP_SHL_Communication_Loop_State."Idle" ("Action") WSVCAP_SHL_Communication_Loop_State."Pre-Transmission" ("Action")] -> w47
          tunnel: w46 -> [w49 w71]
          tunnel: [w49 w72] -> w45
          tunnel: "Wait Ticks" -> [_ w58]
          tunnel: "Slave Address" -> [_ w56]
          tunnel: "Sub Address" -> [_ w70]
          tunnel: "Display CH (1-48)" -> [_ w68]
          tunnel: "Transaction" -> [_ w61]
          tunnel: "Bytes to Write" -> [_ w57]
          tunnel: "Bytes to Read" -> [_ w53]
          tunnel: "Socket Mask" -> [_ w69]
          tunnel: "UUT Set" -> [_ w54]
          frame "Idle" {
            # "This Case Should not Happen"
          }
          frame "Transfer Data" {
            w55 = FALSE ("Read Flag")
            w59 = TRUE ("Read Flag")
            # "Load Transfer State Machine Cluster"
            n19 = case shown="\"RFFE-Ext Write\"" w61 {
              tunnel: [WSVCAP_SHL_Transaction_Step_Enum."I2C Write - I:Send Slave Address" ("Transaction Step") WSVCAP_SHL_Transaction_Step_Enum."RFFE Ext Write - I.Write Data" ("Transaction Step") WSVCAP_SHL_Transaction_Step_Enum."RFFE Ext Read - I:Read Data" ("Transaction Step") WSVCAP_SHL_Transaction_Step_Enum."I2C Read - I:Send Slave Address (W)" ("Transaction Step")] -> w60
              frame "I2C-Write Data" {
              }
              frame "RFFE-Ext Write" {
              }
              frame "RFFE-Ext Read" {
              }
              frame "I2C-Read Data" {
              }
            }
            n20 = disable-structure shown="TARGET_TYPE==FPGA, Default" {
              disable-tunnel: w68 -> [w78 _]
              frame condition #0 (active) {
                n21 = global write "WSVCAP SHL FPGA LL RFFE Debug Global.vi" "RFFE CH (1-16)"(w78) -> ()
                n22 = global write "WSVCAP SHL FPGA LL I2C Debug Global.vi" "I2C CH (1-32)"(w78) -> ()
              }
              frame condition #1 {
              }
            }
            n23 = local write "Read Flag"(w55) -> ()
            n24 = local write "Read Status Flag"(w55) -> ()
            n25 = Logical Shift(y=u8 3, x=w53) -> (x << y=w51:u8)
            n26 = Bundle By Name(cluster=w71, "UUT Set (0/1)"=w54, "Wait Ticks"=w58, "Read Bits Remaining"=w51, "Transaction"=w61, "Bytes to Write"=w57, "Bytes to Read"=w53, "Sub Address"=w70, "Socket Mask"=w69, "Transaction Step"=w60, "Slave Address"=w56, "Operation Step"=WSVCAP_SHL_Operation_Step_Enum."I2C Send Slave Add - A: Send Start Sequence", "Procedure Step"=WSVCAP_SHL_Procedure_Step_Enum."I2C Start/Stop - 1: Set Clock Low", "Write CMD [1-4]"=u8 0, "Write Bit Index [0-39]"=u8 0, "Cycle Count"=u64 0 ("SPI Cycle Count"), "Wait Ticks Remaining"=u32 0, "Start Operation"=w59, "Start Procedure"=w59) -> (w72:T11)
          }
        }
      }
      frame "Pre-Transmission" {
        # "1 Second (ms)"
        # "Transfer All Data from Host into Write FIFO / Initialize Transfer State Machine and SPI Bus Data"
        n27 = disable-structure shown="TARGET_TYPE==FPGA, Default" {
          disable-tunnel: [_ i16 0] -> w79
          frame condition #0 (active) {
            n28 = property on="Waveform Chart" class="WFChart (strict)"("History Data"=cluster{i16, i16, i16, i16}[] []) -> ()  [unwired: 2 in, 2 out]
          }
          frame condition #1 {
          }
        }
        n29 = Unbundle By Name(w81) -> ("Bytes to Write"=w89:u8, "Transaction"=w82:T1)
        n30 = case shown="\"I2C-Write Data\"..\"RFFE-Ext Read\"" w82 {
          selector: w82 -> [_ w105]
          tunnel: w89 -> [_ w100]
          tunnel: [w95 w111] -> w83
          tunnel: w88 -> [w95 w110]
          tunnel: w87 -> [_ w109]
          tunnel: w86 -> [_ w108]
          tunnel: w85 -> [w94 w107]
          tunnel: [w94 w106] -> w84
          tunnel: w81 -> [w93 w102]
          tunnel: [w93 w101] -> w80
          tunnel: w79 -> [_ _]
          frame "I2C-Read Data" {
          }
          frame "I2C-Write Data".."RFFE-Ext Read" {
            # "Bits"
            # "Bytes"
            # "Not I2C"
            # "SPI/RFFE Already In Bits\nI2C Bytes to Bits"
            n31 = To Long Integer(number=w100) -> (32bit integer=w98:i32)
            n32 = Greater Or Equal?(x=w105, y=WSVCAP_SHL_Transaction_Enum."RFFE-Ext Write" ("Transaction")) -> (x >= y?=w103:bool)
            n33 = Logical Shift(y=u8 3 ("x"), x=w98) -> (x << y=w97:i32)
            n34 = Select(t=w98, s=w103, f=w97) -> (s? t:f=w99:i32)
            n35 = for {
              N: w99 -> [w112]
              shift-right: [w129] -> w111
              shift-left: w110 -> [w127]
              tunnel: w105 -> [w125]
              tunnel: w109 -> [w123]
              tunnel: w108 -> [w122]
              shift-right: [w120] -> w106
              shift-left: w107 -> [w121]
              shift-right: [w114] -> w101
              shift-left: w102 -> [w115]
              i -> [w117]
              # "Fill up the FIFO/CMD and CMD Lengths with Write Data from the host"
              n36 = call "Tick Count"() -> ("Tick Count(mSec)"=w124:u32)
              n37 = flat-sequence {
                tunnel: [w138] -> w128
                tunnel: w127 -> [w139]
                tunnel: [w145] -> w126
                tunnel: w125 -> [w145]
                tunnel: w124 -> [w144]
                tunnel: w123 -> [w143]
                tunnel: w122 -> [w137]
                tunnel: w121 -> [w136]
                tunnel: [w135] -> w119
                tunnel: [w133] -> w118
                tunnel: w117 -> [w134]
                tunnel: [w132] -> w116
                tunnel: w115 -> [w132]
                tunnel: [w131] -> w113
                tunnel: w112 -> [w131]
                tunnel: [FALSE ("SPI_Write Flag")] -> w130
                tunnel: [w171] -> w129
                tunnel: w128 -> [w170]
                tunnel: w126 -> [w169]
                tunnel: [w168] -> w120
                tunnel: w119 -> [w168]
                tunnel: w118 -> [w167]
                tunnel: w116 -> [w166]
                tunnel: [w165] -> w114
                tunnel: w113 -> [w163]
                frame #0 {
                  n38 = while {
                    tunnel: w144 -> [w160]
                    tunnel: w143 -> [w158]
                    tunnel: w139 -> [w157]
                    tunnel: ["Write Flag"] -> w142
                    tunnel: [w153] -> w141
                    stop <- w155 stop-if-true
                    n39 = Unbundle By Name(w157) -> ("status"=w156:bool)
                    n40 = call "Wait"("Count(mSec)"=u32 1 ("Count(Ticks)")) -> ("Tick Count(mSec)"=w161:u32)
                    n41 = Subtract(x=w161, y=w160) -> (x-y=w159:u32)
                    n42 = Greater?(x=w159, y=w158) -> (0:w153:bool)
                    n43 = Compound Arithmetic op=OR(w156, w153, "Write Flag") -> (w155:bool)
                  }
                  n44 = To Unsigned Long Integer(number=w134) -> (unsigned 32bit integer=w133:u32)
                  n45 = Compound Arithmetic op=AND(w141, invert w142) -> (w140:bool)
                  n46 = case shown="True" w140 {
                    selector: w140 -> [_ w151]
                    tunnel: [w147 w150] -> w138
                    tunnel: w139 -> [w147 w152]
                    tunnel: w137 -> [_ w148]
                    tunnel: [w146 w148] -> w135
                    tunnel: w136 -> [w146 _]
                    frame False {
                    }
                    frame True {
                      n47 = Bundle By Name(cluster=w152, "status"=w151, "code"=9901) -> (w150:errorcluster)
                    }
                  }
                }
                frame #1 {
                  n48 = case shown="\"RFFE-Ext Write\", \"RFFE-Ext Read\"" w169 {
                    tunnel: "Write Data" -> [w173 w182 _]
                    tunnel: [w176 w183 w276] -> w171
                    tunnel: w170 -> [w175 w184 w276]
                    tunnel: w167 -> [_ w185 _]
                    tunnel: w166 -> [w174 w180 w275]
                    tunnel: [w174 w181 w275] -> w165
                    tunnel: w163 -> [_ w178 _]
                    frame "I2C-Write Data" {
                      n49 = call "WSVCAP SHL FPGA LL I2C FIFO Manager - Pre and Post.vi"("64 Bit Data In"=w173, "error in (no error)"=w175, "Operation"=WSVCAP_SHL_FIFO_Operation_Enum."Put Element in Write") -> ("error out"=w176:errorcluster)  [unwired: 10 in, 2 out]
                    }
                    frame "RFFE-Ext Write", "RFFE-Ext Read" {
                      # "Iteration"
                      n50 = Unbundle By Name(w180) -> ("Cycle Mode"=w179:bool)
                      n51 = case shown="0" w185 {
                        selector: w185 -> [w187 _ _ _ _ _ _ _ _ _]
                        tunnel: w184 -> [w192 w229 w237 w242 w247 w252 w257 w262 w267 w272]
                        tunnel: [w191 w229 w237 w242 w247 w252 w257 w262 w267 w272] -> w183
                        tunnel: w182 -> [w190 w231 w236 w241 w246 w251 w256 w261 w266 w271]
                        tunnel: w180 -> [w189 w228 w239 w244 w249 w254 w259 w264 w269 w274]
                        tunnel: [w188 w230 w238 w243 w248 w253 w258 w263 w268 w273] -> w181
                        tunnel: w179 -> [w186 _ _ _ _ _ _ _ _ _]
                        tunnel: w178 -> [_ w224 _ _ _ _ _ _ _ _]
                        frame Default {
                          # "RFFE Write Data"
                          n52 = case shown="False" w186 {
                            tunnel: w192 -> [w198 w200]
                            tunnel: [w197 w200] -> w191
                            tunnel: w190 -> [w193 w199]
                            tunnel: w189 -> [w194 w203]
                            tunnel: [w194 w202] -> w188
                            tunnel: w187 -> [_ w201]
                            frame False {
                              n53 = To Unsigned Word Integer(number=w193) -> (unsigned 16bit integer=w195:u16)
                              n54 = call "WSVCAP SHL FPGA LL RFFE FIFO Manager - Pre and Post.vi"("Word In"=w195, "error in (no error)"=w198, "Operation"=WSVCAP_SHL_FIFO_Operation_Enum."Put Element in Write") -> ("error out"=w197:errorcluster)  [unwired: 10 in, 2 out]
                            }
                            frame True {
                              n55 = case shown="..9" w201 {
                                tunnel: [w204 w206 w209 w212 w215] -> w202
                                tunnel: w203 -> [w204 w207 w210 w213 w216]
                                tunnel: w199 -> [_ w205 w208 w211 w214]
                                frame Default {
                                }
                                frame ..9 {
                                n56 = Bundle By Name(cluster=w207, "Cycle CMD"=w205, "CMD 1"=w205) -> (w206:T11)
                                }
                                frame 10 {
                                n57 = Bundle By Name(cluster=w210, "CMD 2"=w208) -> (w209:T11)
                                }
                                frame 11 {
                                n58 = Bundle By Name(cluster=w213, "CMD 3"=w211) -> (w212:T11)
                                }
                                frame 12 {
                                n59 = Bundle By Name(cluster=w216, "CMD 4"=w214) -> (w215:T11)
                                }
                              }
                            }
                          }
                        }
                        frame 0 {
                          n60 = To Unsigned Byte Integer(number=w224) -> (unsigned 8bit integer=w222:u8)
                          n61 = To Unsigned Long Integer(number=w231) -> (unsigned 32bit integer=w227:u32)
                          n62 = Subtract(x=w222, y=u8 9) -> (x-y=w219:u8)
                          n63 = Logical Shift(y=i8 -3, x=w219) -> (x << y=w218:u8)
                          n64 = Greater Than 0?(x=w227) -> (x > 0?=w226:bool)
                          n65 = Max & Min(x=w227, y=u32 1) -> (max(x,y)=w232:u32)  [unwired: 1 out]
                          n66 = Select(t=u8 0, s=w226, f=w218) -> (s? t:f=w221:u8)
                          n67 = To Unsigned Byte Integer(number=w232) -> (unsigned 8bit integer=w234:u8)
                          n68 = Bundle By Name(cluster=w228, "Read Bytes Remaining"=u8 7, "Bytes to Write"=w221, "Cycle Mode"=w226, "Commands per Cycle [1-4]"=w234) -> (w230:T11)
                        }
                        frame 1 {
                          n69 = To Unsigned Byte Integer(number=w236) -> (unsigned 8bit integer=w235:u8)
                          n70 = Bundle By Name(cluster=w239, "CMD Length [1-48]"=w235, "CMD 1 Length (Bits)"=w235) -> (w238:T11)
                        }
                        frame 2 {
                          n71 = To Unsigned Byte Integer(number=w241) -> (unsigned 8bit integer=w240:u8)
                          n72 = Bundle By Name(cluster=w244, "CMD 2 Length (Bits)"=w240) -> (w243:T11)
                        }
                        frame 3 {
                          n73 = To Unsigned Byte Integer(number=w246) -> (unsigned 8bit integer=w245:u8)
                          n74 = Bundle By Name(cluster=w249, "CMD 3 Length (Bits)"=w245) -> (w248:T11)
                        }
                        frame 4 {
                          n75 = To Unsigned Byte Integer(number=w251) -> (unsigned 8bit integer=w250:u8)
                          n76 = Bundle By Name(cluster=w254, "CMD 4 Length (Bits)"=w250) -> (w253:T11)
                        }
                        frame 5 {
                          n77 = To Unsigned Long Integer(number=w256) -> (unsigned 32bit integer=w255:u32)
                          n78 = Bundle By Name(cluster=w259, "CMD Delay (Ticks)"=w255, "CMD 1 Delay (Ticks)"=w255) -> (w258:T11)
                        }
                        frame 6 {
                          n79 = To Unsigned Long Integer(number=w261) -> (unsigned 32bit integer=w260:u32)
                          n80 = Bundle By Name(cluster=w264, "CMD 2 Delay (Ticks)"=w260) -> (w263:T11)
                        }
                        frame 7 {
                          n81 = To Unsigned Long Integer(number=w266) -> (unsigned 32bit integer=w265:u32)
                          n82 = Bundle By Name(cluster=w269, "CMD 3 Delay (Ticks)"=w265) -> (w268:T11)
                        }
                        frame 8 {
                          n83 = To Unsigned Long Integer(number=w271) -> (unsigned 32bit integer=w270:u32)
                          n84 = Bundle By Name(cluster=w274, "CMD 4 Delay (Ticks)"=w270) -> (w273:T11)
                        }
                      }
                    }
                    frame "I2C-Read Data" {
                      # "Can't Happen"
                    }
                  }
                }
              }
              n85 = local write "Write Flag"(w130) -> ()
            }
          }
        }
      }
      frame "Transmit Data" {
        # "Perform Write/Read Operation for All Bytes"
        n86 = node-c288() -> (w283:T8)  [unwired: 1 out]
        n87 = timed-loop {
          timing-out: [_] -> w282
          timing: w283 -> [_]
          shift-right: [w310] -> w280
          shift-left: w281 -> [w318]
          tunnel: w279 -> [w315]
          tunnel: [w312] -> w278
          tunnel: [w322] -> w277
          stop <- w323 stop-if-true
          # "LD CMD"
          # "Transaction"
          # "Transaction"
          # "Transaction Finished"
          # "Procedure Finished"
          # "Next Operation Step"
          # "Operation Finished"
          # "Procedure Finished"
          # "Operation Finished"
          # "Next Operation Step"
          # "Procedure Finished"
          # "Operation Step"
          # "Cycle Mode"
          # "CMD Delay (Ticks)"
          # "Transaction Step"
          n88 = call "WSVCAP SHL FPGA LL Manage Initial States.vi"("Transfer Cluster In"=w318) -> ("Transfer Cluster Out"=w316:T11)  [unwired: 14 in]
          n89 = Unbundle By Name(w316) -> ("Transaction"=w320:T1, "Transaction Step"=w319:T7, "Procedure"=w317:T12, "Bytes to Read"=w287:u8, "CMD Length [1-48]"=w295:u8, "CMD Delay (Ticks)"=w294:u32, "Start Procedure"=w305:bool, "Wait Ticks Remaining"=w304:u32, "Procedure Step"=w303:T5, "Wait Ticks"=w302:u32, "Write Bits Remaining"=w301:u8, "Write Byte"=w300:u8, "Read Bits Remaining"=w298:u8, "Read Bytes Remaining"=w286:u8, "Write Bit Index [0-39]"=w296:u8, "Cycle Mode"=w293:bool, "Cycle CMD"=w297:u64, "Socket Mask"=w299:u64, "Operation Step"=w288:T6, "Write CMD [1-4]"=w289:u8, "Commands per Cycle [1-4]"=w290:u8, "UUT Set (0/1)"=w285:u8)
          n90 = case "Execute Procedure" shown="\"I2C-Send Address Byte\"" w317 {
            tunnel: w315 -> [w482 w498 w513 w527 w539 w555 w569 w586 w596 w608 w623 w640]
            tunnel: [w482 w497 w512 w526 w538 w554 w568 w585 w595 w607 w622 w639] -> w314
            tunnel: [TRUE ("Finished") w496 w506 w525 w537 w549 w567 w572 TRUE ("Finished") w599 w609 w630] -> w307
            tunnel: w316 -> [w483 w493 w511 w524 w535 w553 w561 w580 w594 w606 w621 w638]
            tunnel: [w483 w494 w510 w523 w536 w552 w560 w579 w593 w605 w620 w637] -> w292
            tunnel: w294 -> [_ _ _ _ _ _ _ w581 _ _ _ _]
            tunnel: w305 -> [_ _ _ _ _ _ _ w573 _ _ _ w626]
            tunnel: w304 -> [_ w489 w508 w519 w530 w551 w564 w583 _ w602 w616 w633]
            tunnel: w303 -> [_ w491 w504 w518 w533 w545 w563 _ _ w603 w617 w634]
            tunnel: w302 -> [_ w487 w503 w517 w532 w544 w562 _ _ w598 w611 w628]
            tunnel: w299 -> [_ w486 w500 w515 w531 w541 w565 _ _ w604 _ w636]
            tunnel: w301 -> [_ _ w502 w516 _ _ _ _ _ _ _ _]
            tunnel: w300 -> [_ _ w501 _ _ _ _ _ _ _ _ _]
            tunnel: w298 -> [_ _ _ _ _ w543 _ _ _ _ _ w627]
            tunnel: w286 -> [_ _ _ _ _ w542 w557 _ _ _ _ w625]
            tunnel: w297 -> [_ _ _ _ _ _ _ _ _ _ w619 w635]
            tunnel: w293 -> [_ _ _ _ _ _ _ _ w592 _ w618 _]
            tunnel: w296 -> [_ _ _ _ _ _ _ _ _ _ w610 _]
            tunnel: w295 -> [_ _ _ _ _ _ _ _ _ _ w615 _]
            tunnel: "Stop Cycle" -> [_ _ _ _ _ _ _ w570 w591 _ _ _]
            tunnel: w290 -> [_ _ _ _ _ _ _ w577 _ _ _ _]
            tunnel: w289 -> [_ _ _ _ _ _ _ w575 _ _ _ _]
            tunnel: w288 -> [_ w485 _ _ _ _ _ _ _ _ _ _]
            tunnel: w287 -> [_ _ _ _ _ _ _ _ _ _ _ _]
            tunnel: w285 -> [_ w484 w499 w514 w528 w540 w556 _ _ _ _ _]
            frame "None" {
            }
            frame "I2C-Send Start/Stop Sequence" {
              n91 = Equal?(x=w485, y=WSVCAP_SHL_Operation_Step_Enum."I2C Send Slave Add - A: Send Start Sequence" ("Operation Step")) -> (x = y?=w492:bool)
              n92 = call "WSVCAP SHL FPGA LL Procedure I2C - Send Start or Stop Sequence.vi"("Procedure Step"=w491, "Wait Ticks Remaining"=w489, "I2C Wait Ticks"=w487, "error in (no error)"=w498, "Type (T:Start; F:Stop)"=w492, "Socket Mask"=w486, "UUT Set (0/1)"=w484) -> ("Wait Ticks Remaining Out"=w488:u32, "Procedure Step Out"=w490:T5, "Finished"=w496:bool, "error out"=w497:errorcluster)  [unwired: 5 in]
              n93 = Bundle By Name(cluster=w493, "Wait Ticks Remaining"=w488, "Procedure Step"=w490) -> (w494:T11)
            }
            frame "I2C-Send Address Byte" {
              n94 = call "WSVCAP SHL FPGA LL Procedure I2C - Send Address Byte.vi"("Procedure Step"=w504, "Wait Ticks Remaining"=w508, "I2C Wait Ticks"=w503, "Write Bits Remaining"=w502, "Write Byte"=w501, "error in (no error)"=w513, "Socket Mask"=w500, "UUT Set (0/1)"=w499) -> ("Wait Ticks Remaining Out"=w507:u32, "Procedure Step Out"=w509:T5, "Write Bits Remaining Out"=w505:u8, "Finished"=w506:bool, "error out"=w512:errorcluster)  [unwired: 3 in]
              n95 = Bundle By Name(cluster=w511, "Wait Ticks Remaining"=w507, "Procedure Step"=w509, "Write Bits Remaining"=w505) -> (w510:T11)
            }
            frame "I2C-Send Data Byte" {
              n96 = call "WSVCAP SHL FPGA LL I2C Procedure - Send Data Byte.vi"("Procedure Step"=w518, "Wait Ticks Remaining"=w519, "I2C Wait Ticks"=w517, "Write Bits Remaining"=w516, "error in (no error)"=w527, "Socket Mask"=w515, "UUT (0/1)"=w514) -> ("Wait Ticks Remaining Out"=w522:u32, "Procedure Step Out"=w521:T5, "Write Bits Remaining Out"=w520:u8, "Finished"=w525:bool, "error out"=w526:errorcluster)  [unwired: 4 in]
              n97 = Bundle By Name(cluster=w524, "Wait Ticks Remaining"=w522, "Procedure Step"=w521, "Write Bits Remaining"=w520) -> (w523:T11)
            }
            frame "I2C-Read ACK" {
              n98 = call "WSVCAP SHL FPGA LL Procedure I2C - Read ACK.vi"("Procedure Step"=w533, "Wait Ticks Remaining"=w530, "I2C Wait Ticks"=w532, "Socket Mask"=w531, "error in (no error)"=w539, "UUT Set (0/1)"=w528) -> ("Wait Ticks Remaining Out"=w529:u32, "Procedure Step Out"=w534:T5, "Finished"=w537:bool, "error out"=w538:errorcluster)  [unwired: 5 in, 1 out]
              n99 = Bundle By Name(cluster=w535, "Wait Ticks Remaining"=w529, "Procedure Step"=w534) -> (w536:T11)
            }
            frame "I2C-Receive Byte" {
              n100 = call "WSVCAP SHL FPGA LL Procedure I2C - Receive Byte.vi"("Procedure Step"=w545, "Wait Ticks Remaining"=w551, "I2C Wait Ticks"=w544, "Read Bits Remaining"=w543, "Read Bytes Remaining"=w542, "error in (no error)"=w555, "Socket Mask"=w541, "UUT Set (0/1)"=w540) -> ("Wait Ticks Remaining Out"=w550:u32, "Procedure Step Out"=w548:T5, "Finished"=w549:bool, "Read Bits Remaining Out"=w547:u8, "Read Bytes Remaining Out"=w546:u8, "error out"=w554:errorcluster)  [unwired: 2 in]
              n101 = Bundle By Name(cluster=w553, "Wait Ticks Remaining"=w550, "Procedure Step"=w548, "Read Bits Remaining"=w547, "Read Bytes Remaining"=w546) -> (w552:T11)
            }
            frame "I2C-Write ACK" {
              n102 = Less Or Equal To 0?(x=w557) -> (x <= 0?=w566:bool)
              n103 = call "WSVCAP SHL FPGA LL Procedure I2C - Send ACK.vi"("Procedure Step"=w563, "Wait Ticks Remaining"=w564, "I2C Wait Ticks"=w562, "ACK Bit to Write"=w566, "error in (no error)"=w569, "Socket Mask"=w565, "UUT (0/1)"=w556) -> ("Wait Ticks Remaining Out"=w559:u32, "Procedure Step Out"=w558:T5, "Finished"=w567:bool, "error out"=w568:errorcluster)  [unwired: 5 in]
              n104 = Bundle By Name(cluster=w561, "Wait Ticks Remaining"=w559, "Procedure Step"=w558) -> (w560:T11)
            }
            frame "RFFE-Wait CMD Delay" {
              # "Last Tick"
              # "First Tick"
              n105 = Select(t=w581, s=w573, f=w583) -> (s? t:f=w582:u32)
              n106 = Equal?(x=w575, y=w577) -> (x = y?=w576:bool)
              n107 = Decrement(x=w582) -> (x-1=w584:u32)
              n108 = Compound Arithmetic op=AND(w576, w570) -> (w574:bool)
              n109 = Less Or Equal To 0?(x=w584) -> (x <= 0?=w572:bool)
              n110 = Compound Arithmetic op=AND(w572, invert w574) -> (w571:bool)
              n111 = Compound Arithmetic op=OR(w571, w573) -> (w578:bool)
              n112 = Bundle By Name(cluster=w580, "Wait Ticks Remaining"=w584) -> (w579:T11)
              n113 = case shown="True" w578 {
                tunnel: w586 -> [w587 w589]
                tunnel: [w587 w588] -> w585
                frame False {
                }
                frame True {
                  # "First or Last Tick of Wait Cycle"
                  n114 = call "WSVCAP SHL FPGA LL Procedure RFFE - Clear Lines.vi"("error in (no error)"=w589) -> ("error out"=w588:errorcluster)  [unwired: 14 in]
                }
              }
            }
            frame "RFFE-Clear Lines" {
              n115 = Compound Arithmetic op=AND(w592, invert w591) -> (w590:bool)
              n116 = Bundle By Name(cluster=w594, "Cycle Mode"=w590) -> (w593:T11)
              n117 = call "WSVCAP SHL FPGA LL Procedure RFFE - Clear Lines.vi"("error in (no error)"=w596) -> ("error out"=w595:errorcluster)  [unwired: 14 in]
            }
            frame "RFFE-Send SSC" {
              n118 = call "WSVCAP SHL FPGA LL Procedure RFFE - Send SSC.vi"("Procedure Step"=w603, "Wait Ticks Remaining"=w602, "Wait Ticks"=w598, "error in (no error)"=w608, "Socket Mask"=w604) -> ("Wait Ticks Remaining Out"=w601:u32, "Procedure Step Out"=w600:T5, "Finished"=w599:bool, "error out"=w607:errorcluster)  [unwired: 7 in]
              n119 = Bundle By Name(cluster=w606, "Wait Ticks Remaining"=w601, "Procedure Step"=w600) -> (w605:T11)
            }
            frame "RFFE-Send Data" {
              n120 = call "WSVCAP SHL FPGA LL Procedure RFFE - Send Data.vi"("Procedure Step"=w617, "Wait Ticks Remaining"=w616, "CMD Length [1-48]"=w615, "RFFE Wait Ticks"=w611, "Write Bit Index [0-47]"=w610, "RFFE Cycle Mode"=w618, "error in (no error)"=w623, "RFFE Cycle CMD"=w619) -> ("Wait Ticks Remaining Out"=w614:u32, "Procedure Step Out"=w613:T5, "Write Bit Index [0-47] Out"=w612:u8, "Finished"=w609:bool, "error out"=w622:errorcluster)  [unwired: 3 in]
              n121 = Bundle By Name(cluster=w621, "Wait Ticks Remaining"=w614, "Procedure Step"=w613, "Write Bit Index [0-39]"=w612) -> (w620:T11)
            }
            frame "RFFE-Receive Data" {
              n122 = call "WSVCAP SHL FPGA LL Procedure RFFE - Receive Data.vi"("Procedure Step"=w634, "Wait Ticks Remaining"=w633, "Start of Procedure"=w626, "RFFE Wait Ticks"=w628, "Read Bits Remaining"=w627, "Read Bytes Remaining"=w625, "error in (no error)"=w640, "RFFE Cycle CMD"=w635, "Socket Mask"=w636) -> ("Wait Ticks Remaining Out"=w632:u32, "Procedure Step Out"=w631:T5, "Read Bytes Remaining Out"=w624:u8, "Read Bits Remaining Out"=w629:u8, "Finished"=w630:bool, "error out"=w639:errorcluster)  [unwired: 1 in]
              n123 = Bundle By Name(cluster=w638, "Wait Ticks Remaining"=w632, "Procedure Step"=w631, "Read Bytes Remaining"=w624, "Read Bits Remaining"=w629) -> (w637:T11)
            }
          }
          n124 = case "Post-Procedure" shown="\"I2C Send Data - B: Send Data Byte\"" w288 {
            selector: w288 -> [w363 w366 w371 w372 w376 w380 w383 _ w390 w403 w404 w408 w410 w420 w424 w430 w435 w438 w443 w461 w476 w479]
            tunnel: [w361 w365 w369 w373 w377 w382 w385 w387 w392 w399 w406 w409 w414 w423 w426 w432 w437 w440 w445 w465 w477 w480] -> w312
            tunnel: w314 -> [w361 w365 w369 w373 w377 w382 w385 w387 w392 w400 w406 w409 w414 w423 w426 w432 w437 w440 w445 w465 w477 w480]
            tunnel: [_ _ _ w374 _ _ w384 _ _ _ w405 _ _ _ w425 _ _ w439 _ _ _ w478] -> w306
            tunnel: w307 -> [w360 _ w368 w374 _ w379 w384 _ w388 w401 w405 _ w412 w422 w425 w429 w433 w439 w441 w455 w469 w478]
            tunnel: [w359 w364 w367 w372 w375 w378 w383 WSVCAP_SHL_Operation_Step_Enum."I2C Send Data - B: Send Data Byte" ("Operation Step") w389 w402 w404 w407 w411 w421 w424 w428 w434 w438 w442 w464 w475 w479] -> w308
            tunnel: [_ _ _ _ _ _ _ _ _ _ _ _ _ _ _ TRUE ("Finished") _ _ w441 w456 _ _] -> w313
            tunnel: w294 -> [_ _ _ _ _ _ _ _ _ _ _ _ _ _ _ _ _ _ _ w452 _ _]
            tunnel: w293 -> [_ _ _ _ _ _ _ _ _ _ _ _ _ _ _ _ _ _ _ w454 _ _]
            tunnel: "Stop Cycle" -> [_ _ _ _ _ _ _ _ _ _ _ _ _ _ _ _ _ _ _ w446 w468 _]
            tunnel: w289 -> [_ _ _ _ _ _ _ _ _ _ _ _ _ _ _ _ _ _ _ w451 w471 _]
            tunnel: w290 -> [_ _ _ _ _ _ _ _ _ _ _ _ _ _ _ _ _ _ _ w450 w470 _]
            tunnel: w286 -> [_ _ _ _ _ _ _ _ _ _ _ _ _ w415 _ _ _ _ _ _ _ _]
            frame "I2C Send Slave Add - A: Send Start Sequence" {
              n125 = Increment(x=w363) -> (x+1=w362:T6)
              n126 = Select(t=w362, s=w360, f=w363) -> (s? t:f=w359:T6)
            }
            frame "I2C Send Slave Add - B: Load Address Byte" {
              n127 = Increment(x=w366) -> (x+1=w364:T6)
            }
            frame "I2C Send Slave Add - C: Send Address Byte" {
              n128 = Increment(x=w371) -> (x+1=w370:T6)
              n129 = Select(t=w370, s=w368, f=w371) -> (s? t:f=w367:T6)
            }
            frame "I2C Send Slave Add - D: Read Slave ACK" {
            }
            frame "I2C Send Sub Add - A: Load Sub Address" {
              n130 = Increment(x=w376) -> (x+1=w375:T6)
            }
            frame "I2C Send Sub Add - B: Send Address Byte" {
              n131 = Increment(x=w380) -> (x+1=w381:T6)
              n132 = Select(t=w381, s=w379, f=w380) -> (s? t:f=w378:T6)
            }
            frame "I2C Send Sub Add - C: Read Slave ACK" {
            }
            frame "I2C Send Data - A: Get Byte from FIFO" {
            }
            frame "I2C Send Data - B: Send Data Byte" {
              n133 = Increment(x=w390) -> (x+1=w391:T6)
              n134 = Select(t=w391, s=w388, f=w390) -> (s? t:f=w389:T6)
            }
            frame "I2C Send Data - C: Read Slave ACK" {
              n135 = call "WSVCAP SHL FPGA LL I2C FIFO Manager - Transfer.vi"("error in (no error)"=w400, "Operation"=WSVCAP_SHL_FIFO_Operation_Enum."Get Write FIFO Status") -> ("Data Out"=w397:u64, "error out"=w399:errorcluster)  [unwired: 11 in, 1 out]
              n136 = Equal To 0?(x=w397) -> (x = 0?=w396:bool)
              n137 = Select(t=WSVCAP_SHL_Operation_Step_Enum."I2C Send Data - D: Send Stop Sequence" ("Operation Step"), s=w396, f=WSVCAP_SHL_Operation_Step_Enum."I2C Send Data - A: Get Byte from FIFO" ("Operation Step")) -> (s? t:f=w393:T6)
              n138 = Select(t=w393, s=w401, f=w403) -> (s? t:f=w402:T6)
            }
            frame "I2C Send Data - D: Send Stop Sequence" {
            }
            frame "I2C Read Data - A: Load Bytes to Read" {
              n139 = Increment(x=w408) -> (x+1=w407:T6)
            }
            frame "I2C Read Data - B: Receive Byte" {
              n140 = Increment(x=w410) -> (x+1=w413:T6)
              n141 = Select(t=w413, s=w412, f=w410) -> (s? t:f=w411:T6)
            }
            frame "I2C Read Data - C: Write Master ACK" {
              n142 = Less Or Equal To 0?(x=w415) -> (x <= 0?=w416:bool)
              n143 = Increment(x=w420) -> (x+1=w418:T6)
              n144 = Select(t=w418, s=w416, f=WSVCAP_SHL_Operation_Step_Enum."I2C Read Data - B: Receive Byte" ("Operation Step")) -> (s? t:f=w417:T6)
              n145 = Select(t=w417, s=w422, f=w420) -> (s? t:f=w421:T6)
            }
            frame "I2C Read Data - D: Send Stop Sequence" {
            }
            frame "RFFE Read Data - A: Send SSC" {
              n146 = Increment(x=w430) -> (x+1=w431:T6)
              n147 = Select(t=w431, s=w429, f=w430) -> (s? t:f=w428:T6)
            }
            frame "RFFE Read Data - B: Send CMD Frame" {
              n148 = Increment(x=w435) -> (x+1=w436:T6)
              n149 = Select(t=w436, s=w433, f=w435) -> (s? t:f=w434:T6)
            }
            frame "RFFE Read Data - C: Receive Byte" {
            }
            frame "RFFE Write Data - A: Send SSC" {
              n150 = Increment(x=w443) -> (x+1=w444:T6)
              n151 = Select(t=w444, s=w441, f=w443) -> (s? t:f=w442:T6)
            }
            frame "RFFE Write Data - B: Send Data" {
              n152 = Equal To 0?(x=w452) -> (x = 0?=w447:bool)
              n153 = Equal?(x=w451, y=w450) -> (x = y?=w449:bool)
              n154 = Compound Arithmetic op=AND(w449, w446) -> (w448:bool)
              n155 = Select(t=WSVCAP_SHL_Operation_Step_Enum."RFFE Write Data - A: Send SSC" ("Operation Step"), s=w447, f=WSVCAP_SHL_Operation_Step_Enum."RFFE Write Data - C: Wait CMD Delay" ("Operation Step")) -> (s? t:f=w458:T6)
              n156 = Select(t=WSVCAP_SHL_Operation_Step_Enum."RFFE Write Data - D: Clear Lines" ("Operation Step"), s=w448, f=w458) -> (s? t:f=w457:T6)
              n157 = Select(t=w457, s=w454, f=WSVCAP_SHL_Operation_Step_Enum."RFFE Write Data - D: Clear Lines" ("Operation Step")) -> (s? t:f=w463:T6)
              n158 = Compound Arithmetic op=AND(w448, w454, w455) -> (w456:bool)
              n159 = Select(t=w463, s=w455, f=w461) -> (s? t:f=w464:T6)
            }
            frame "RFFE Write Data - C: Wait CMD Delay" {
              n160 = Equal?(x=w471, y=w470) -> (x = y?=w467:bool)
              n161 = Compound Arithmetic op=AND(w467, w468) -> (w466:bool)
              n162 = Select(t=WSVCAP_SHL_Operation_Step_Enum."RFFE Write Data - D: Clear Lines" ("f"), s=w466, f=WSVCAP_SHL_Operation_Step_Enum."RFFE Write Data - A: Send SSC") -> (s? t:f=w473:T6)
              n163 = Select(t=w473, s=w469, f=w476) -> (s? t:f=w475:T6)
            }
            frame "RFFE Write Data - D: Clear Lines" {
            }
          }
          n164 = case shown="True" w313 {
            tunnel: w292 -> [w355 w358]
            tunnel: [w355 w357] -> w311
            frame False {
            }
            frame True {
              # "Load next RFFE\nCycle CMD"
              n165 = call "WSVCAP SHL FPGA LL RFFE Load Next Cycle CMD.vi"("Transfer Cluster In"=w358) -> ("Transfer Cluster Out"=w357:T11, "SPI Cycle Count"=→"Cycle Count":u64)  [unwired: 13 in]
            }
          }
          n166 = case "Post Operation" shown="\"I2C Read - II:Send Sub Address\"" w319 {
            selector: w319 -> [w327 w331 w334 w337 w341 w345 w350 w352 w354]
            tunnel: [_ _ w333 _ _ _ w349 w351 w353] -> w321
            tunnel: w306 -> [w325 w329 w333 w336 w340 w344 w349 w351 w353]
            tunnel: [w328 w332 w334 w335 w339 w343 w347 w352 w354] -> w309
            frame "I2C Write - I:Send Slave Address" {
              n167 = Increment(x=w327) -> (x+1=w326:T7)
              n168 = Select(t=w326, s=w325, f=w327) -> (s? t:f=w328:T7)
            }
            frame "I2C Write - II:Send Sub Address" {
              n169 = Increment(x=w331) -> (x+1=w330:T7)
              n170 = Select(t=w330, s=w329, f=w331) -> (s? t:f=w332:T7)
            }
            frame "I2C Write - III:Send Data Bytes" {
            }
            frame "I2C Read - I:Send Slave Address (W)" {
              n171 = Increment(x=w337) -> (x+1=w338:T7)
              n172 = Select(t=w338, s=w336, f=w337) -> (s? t:f=w335:T7)
            }
            frame "I2C Read - II:Send Sub Address" {
              n173 = Increment(x=w341) -> (x+1=w342:T7)
              n174 = Select(t=w342, s=w340, f=w341) -> (s? t:f=w339:T7)
            }
            frame "I2C Read - III:Send Slave Address (R)" {
              n175 = Increment(x=w345) -> (x+1=w346:T7)
              n176 = Select(t=w346, s=w344, f=w345) -> (s? t:f=w343:T7)
            }
            frame "I2C Read - IV:Read Data Bytes" {
              n177 = Select(t=WSVCAP_SHL_Transaction_Step_Enum."I2C Read - I:Send Slave Address (W)" ("Transaction Step"), s=w349, f=w350) -> (s? t:f=w347:T7)
            }
            frame "RFFE Ext Write - I.Write Data" {
            }
            frame "RFFE Ext Read - I:Read Data" {
            }
          }
          n178 = Bundle By Name(cluster=w311, "Transaction Step"=w309, "Operation Step"=w308, "Start Operation"=w306, "Start Procedure"=w307) -> (w310:T11)
          n179 = disable-structure shown="TARGET_TYPE!=FPGA, Default" {
            disable-tunnel: w320 -> [w641 _]
            disable-tunnel: w321 -> [_ _]
            frame condition #0 (active) {
              n180 = case shown="Default" w641 {
                tunnel: [w648 w657] -> w642
                frame "RFFE-Ext Write", "RFFE-Ext Read" {
                  n181 = global read "WSVCAP SHL FPGA LL RFFE Debug Global.vi" "RFFE_CLK"() -> (w647:bool)
                  n182 = global read "WSVCAP SHL FPGA LL RFFE Debug Global.vi" "RFFE_DAA"() -> (w646:bool)
                  n183 = global read "WSVCAP SHL FPGA LL RFFE Debug Global.vi" "RFFE_CLK"() -> (w651:bool)
                  n184 = global read "WSVCAP SHL FPGA LL RFFE Debug Global.vi" "RFFE_DATO"() -> (w644:bool)
                  n185 = Boolean To (0,1)(Boolean=w647) -> (0, 1=w653:i16)
                  n186 = Boolean To (0,1)(Boolean=w646) -> (0, 1=w652:i16)
                  n187 = Boolean To (0,1)(Boolean=w651) -> (0, 1=w645:i16)
                  n188 = Boolean To (0,1)(Boolean=w644) -> (0, 1=w643:i16)
                  n189 = Bundle(w653, w652, w645, w643) -> (w650:cluster{i16, i16, i16, i16})  [unwired: 1 in]
                  n190 = Add(x=w650, y=cluster{i16, i16, i16, i16} {0, 2, 4, 6} ("Waveform Chart")) -> (x+y=w648:cluster{i16, i16, i16, i16})
                }
                frame Default {
                  w656 = i16 0 ("0, 1")
                  n191 = global read "WSVCAP SHL FPGA LL I2C Debug Global.vi" "I2C SCL"() -> (w655:bool)
                  n192 = global read "WSVCAP SHL FPGA LL I2C Debug Global.vi" "I2C SDA"() -> (w654:bool)
                  n193 = Boolean To (0,1)(Boolean=w655) -> (0, 1=w661:i16)
                  n194 = Boolean To (0,1)(Boolean=w654) -> (0, 1=w660:i16)
                  n195 = Bundle(w661, w660, "0, 1"=w656, "0, 1"=w656) -> (w659:cluster{i16, i16, "0, 1":i16, "0, 1":i16})  [unwired: 1 in]
                  n196 = Add(x=w659, y=cluster{i16, i16, i16, i16} {0, 2, -1, -1} ("Waveform Chart")) -> (x+y=w657:cluster{i16, i16, i16, i16})
                }
              }
              "Waveform Chart" <- w642
            }
            frame condition #1 {
            }
          }
          n197 = Unbundle By Name(w312) -> ("status"=w324:bool)
          n198 = To Long Integer(number=w320) -> (32bit integer=w322:i32)
          n199 = Compound Arithmetic op=OR(w321, w324) -> (w323:bool)
        }
        n200 = node-c288(w282) -> ()
      }
      frame "Post Transmition" {
        # "1 Second (Ticks)"
        # "Error Info"
        # "Transfer Data from Read FIFO to Host"
        n201 = Unbundle By Name(w670) -> ("Cycle Count"=w667:u64, "Cycle Mode"=w668:bool, "Bytes to Read"=w672:u8, "Transaction"=w676:T1)
        n202 = Increment(x=w667) -> (x+1=w671:u64)
        n203 = Select(t=w671, s=w668, f=w667) -> (s? t:f=w666:u64)
        n204 = Bundle By Name(cluster=w670, "Cycle Count"=w666) -> (w669:T11)
        n205 = case shown="1.." w672 {
          selector: w672 -> [_ w685]
          tunnel: w678 -> [w681 w691]
          tunnel: [w681 w690] -> w677
          tunnel: w676 -> [_ w689]
          tunnel: w675 -> [_ w688]
          tunnel: [w680 w687] -> w674
          tunnel: w673 -> [w680 w686]
          frame ..0 {
            # "No Read Operation"
          }
          frame 1.. {
            # "Transfer Read Data"
            # "Read all data and transfer to the host"
            n206 = Logical Shift(y=u8 3, x=w685) -> (x << y=w683:u8)
            n207 = To Long Integer(number=w683) -> (32bit integer=w682:i32)
            n208 = for {
              N: w682 -> [_]
              shift-right: [w707] -> w690
              shift-left: w691 -> [w708]
              tunnel: w689 -> [w704]
              tunnel: w688 -> [w703]
              shift-right: [w694] -> w687
              shift-left: w686 -> [w692]
              i -> [w697]
              n209 = flat-sequence {
                tunnel: w708 -> [w715]
                tunnel: [w714] -> w705
                tunnel: w704 -> [w712]
                tunnel: w703 -> [w711]
                tunnel: [w711] -> w702
                tunnel: [w710] -> w698
                tunnel: w697 -> [w710]
                tunnel: [w709] -> w695
                tunnel: w692 -> [w709]
                tunnel: [w728] -> w706
                tunnel: w705 -> [w728]
                tunnel: w702 -> [w727]
                tunnel: [w727] -> w701
                tunnel: [w726] -> w699
                tunnel: w698 -> [w726]
                tunnel: [w725] -> w696
                tunnel: w695 -> [w725]
                tunnel: w706 -> [w737]
                tunnel: w701 -> [w738]
                tunnel: [w736] -> w700
                tunnel: w699 -> [w732]
                tunnel: w696 -> [w731]
                tunnel: [w730] -> w693
                tunnel: [w758] -> w707
                tunnel: w700 -> [w758]
                tunnel: [w757] -> w694
                tunnel: w693 -> [w757]
                frame #0 {
                  n210 = case shown="\"RFFE-Ext Write\", \"RFFE-Ext Read\"" w712 {
                    tunnel: w715 -> [w719 w724]
                    tunnel: [w718 w723] -> w714
                    tunnel: [w717 w720] -> w713
                    frame "I2C-Read Data", "I2C-Write Data" {
                      n211 = call "WSVCAP SHL FPGA LL I2C FIFO Manager - Pre and Post.vi"("error in (no error)"=w719, "Operation"=WSVCAP_SHL_FIFO_Operation_Enum."Get Element from Read") -> ("64 Bit Data Out"=w717:u64, "error out"=w718:errorcluster)  [unwired: 11 in, 1 out]
                    }
                    frame "RFFE-Ext Write", "RFFE-Ext Read" {
                      n212 = call "WSVCAP SHL FPGA LL RFFE FIFO Manager - Pre and Post.vi"("error in (no error)"=w724, "Operation"=WSVCAP_SHL_FIFO_Operation_Enum."Get Element from Read") -> ("Word Out"=w722:u64, "error out"=w723:errorcluster)  [unwired: 11 in, 1 out]
                      n213 = To Unsigned Quad Integer(1:w722) -> (0:w720:u64)
                    }
                  }
                  "Read Data" <- w713
                }
                frame #1 {
                  "Read Flag" <- TRUE ("Read Flag")
                }
                frame #2 {
                  n214 = call "Tick Count2"() -> ("Tick Count(mSec)"=w739:u32)
                  n215 = while {
                    tunnel: w739 -> [w754]
                    tunnel: w738 -> [w752]
                    tunnel: w737 -> [w751]
                    tunnel: ["Ack Read"] -> w734
                    tunnel: [w748] -> w735
                    stop <- w749 stop-if-true
                    n216 = Unbundle By Name(w751) -> ("status"=w750:bool)
                    n217 = call "Wait2"("Count(mSec)"=u32 1 ("Count(Ticks)")) -> ("Tick Count(mSec)"=w755:u32)
                    n218 = Subtract(x=w755, y=w754) -> (x-y=w753:u32)
                    n219 = Greater?(x=w753, y=w752) -> (0:w748:bool)
                    n220 = Compound Arithmetic op=OR(w750, w748, "Ack Read") -> (w749:bool)
                  }
                  n221 = Compound Arithmetic op=AND(w735, invert w734) -> (w733:bool)
                  n222 = case shown="False" w733 {
                    selector: w733 -> [_ w745]
                    tunnel: [w741 w744] -> w736
                    tunnel: w737 -> [w741 w746]
                    tunnel: [w740 w742] -> w730
                    tunnel: w732 -> [_ w742]
                    tunnel: w731 -> [w740 _]
                    frame False {
                    }
                    frame True {
                      n223 = Bundle By Name(cluster=w746, "status"=w745, "code"=9902) -> (w744:errorcluster)
                    }
                  }
                }
                frame #3 {
                  n224 = local write "Ack Read"(FALSE ("Read Flag")) -> ()
                }
              }
            }
          }
        }
      }
      frame "Operation Complete" {
        # "Transfer Status"
        n225 = Unbundle By Name(w761) -> ("Cycle Mode"=w760:bool)
        n226 = To Long Integer(number=w765) -> (32bit integer=w764:i32)
        n227 = case shown="False" w760 {
          tunnel: w766 -> [w773 _]
          tunnel: w764 -> [w772 _]
          tunnel: w763 -> [w771 _]
          tunnel: w762 -> [w769 _]
          frame False {
            # "Return Status"
            n228 = for {
              N: 4 -> [_]
              tunnel: w773 -> [w780]
              tunnel: w772 -> [w779]
              tunnel: w771 -> [w778]
              tunnel: w769 -> [w774]
              i -> [w777]
              n229 = flat-sequence {
                tunnel: w780 -> [w790]
                tunnel: w779 -> [w783]
                tunnel: w778 -> [w782]
                tunnel: w777 -> [w787]
                tunnel: [w781] -> w775
                tunnel: w774 -> [w781]
                tunnel: [w795] -> w776
                tunnel: w775 -> [w795]
                tunnel: w776 -> [w797]
                frame #0 {
                  # "Iteration"
                  # "Error Info"
                  # "Last State"
                  # "Error Code"
                  # "Error Status"
                  n230 = Unbundle By Name(w790) -> ("status"=w789:bool, "code"=w784:i32)
                  n231 = Boolean To (0,1)(Boolean=w789) -> (0, 1=w788:i16)
                  n232 = To Long Integer(number=w788) -> (32bit integer=w786:i32)
                  n233 = case shown="3" w787 {
                    tunnel: [w791 w792 w793 w794] -> w785
                    tunnel: w786 -> [w791 _ _ _]
                    tunnel: w784 -> [_ w792 _ _]
                    tunnel: w783 -> [_ _ w793 _]
                    tunnel: w782 -> [_ _ _ w794]
                    frame Default {
                    }
                    frame 1 {
                    }
                    frame 2 {
                    }
                    frame 3 {
                    }
                  }
                  "Status" <- w785
                }
                frame #1 {
                  "Read Status Flag" <- TRUE ("Read Flag")
                }
                frame #2 {
                  n234 = call "Tick Count3"() -> ("Tick Count(mSec)"=w798:u32)
                  n235 = while {
                    tunnel: w798 -> [w804]
                    tunnel: w797 -> [w802]
                    stop <- w801 stop-if-true
                    n236 = call "Wait3"("Count(mSec)"=u32 1 ("Count(Ticks)")) -> ("Tick Count(mSec)"=w805:u32)
                    n237 = Subtract(x=w805, y=w804) -> (x-y=w803:u32)
                    n238 = Greater?(x=w803, y=w802) -> (0:w800:bool)
                    n239 = Compound Arithmetic op=OR(w800, "Ack Read Status") -> (w801:bool)
                  }
                }
                frame #3 {
                  n240 = local write "Ack Read Status"(FALSE ("Read Flag")) -> ()
                }
              }
            }
          }
          frame True {
            # "No Status from Cycle Mode"
          }
        }
        n241 = local write "Cmd"(WSVCAP_SHL_State."Idle" ("SPI_CMD_DBG")) -> ()
      }
    }
    n242 = Select(t=WSVCAP_SHL_Communication_Loop_State."Operation Complete" ("Action"), s=w19, f=w21) -> (s? t:f=w20:T3)
  }
  n243 = local write "Exit"(w4) -> ()
